vi "Spectrometer Loop.vi"(6 "Used functions":bool, 8 "error in":errorcluster, 9 "Configuration":T1={"Parameter Analizer"={"Parameter Analyzer VISA Session"="COM1", "Sweeping Time Parameters"={"Integration Time"=0, "Short Integration Time (s)"=1.0, "Long Integration Time (s)"=0.0, "Wait Time Parameter"=1.0}, "Acquisition Mode"=enum."Sweeping Mode", "Status Polling Time (ms)"=0, "Comment"="Test VI", "SMU 1 - Sweeping"={"Start / Offset"=0.0, "Stop / Ratio"=1.0, "Step \n(linear only)"=0.01, "Compliance"=0.1, "Power \nCompliance"=0.0, "Mode"=0, "Function"=0, "Sweep Mode"=FALSE}, "SMU 2 - Sweeping"={"Start / Offset"=0.0, "Stop / Ratio"=1.0, "Step \n(linear only)"=0.01, "Compliance"=0.1, "Power \nCompliance"=0.0, "Mode"=0, "Function"=0, "Sweep Mode"=FALSE}, "SMU 3 - Sweeping"={"Start / Offset"=0.0, "Stop / Ratio"=1.0, "Step \n(linear only)"=0.01, "Compliance"=0.1, "Power \nCompliance"=0.0, "Mode"=0, "Function"=0, "Sweep Mode"=FALSE}, "SMU 4 - Sweeping"={"Start / Offset"=0.0, "Stop / Ratio"=1.0, "Step \n(linear only)"=0.01, "Compliance"=0.1, "Power \nCompliance"=0.0, "Mode"=0, "Function"=0, "Sweep Mode"=FALSE}, "Sweep Spacing"=0, "Range"=0, "SMU1 - Sampling"={"Source"=10.0, "Compliance"=1e-05, "Mode"=0, "Function"=FALSE}, "SMU2 - Sampling"={"Source"=1.0, "Compliance"=1.0, "Mode"=0, "Function"=FALSE}, "SMU3 - Sampling"={"Source"=10.0, "Compliance"=1e-05, "Mode"=0, "Function"=FALSE}, "SMU4 - Sampling"={"Source"=0.1, "Compliance"=60.0, "Mode"=10, "Function"=FALSE}, "Sampling Time Parameters"={"Initial Interval (s)"=0.1, "Number of Samples"=60, "Total Sampling Time (s)"=10.0, "Hold Time (s)"=0.0, "Sampling Mode"=0, "Sampling Time"=0}, "Stop Condition"={"Enable Delay (s)"=0.0, "Name"="", "Threshold"=0.0, "num. of events"=1, "Event"=0, "Stop Condition Enable"=FALSE}}, "Switching Matrix"={"Switching Matrix VISA Session"="GPIB0::18::INSTR", "Connections"=[{"Connections"=[FALSE, FALSE, FALSE, FALSE, FALSE, FALSE, FALSE, FALSE, FALSE, FALSE, FALSE, FALSE], "Connection Type"=enum."Disconnected"}, {"Connections"=[FALSE, FALSE, FALSE, FALSE, FALSE, FALSE, FALSE, FALSE, FALSE, FALSE, FALSE, FALSE], "Connection Type"=enum."Disconnected"}, {"Connections"=[FALSE, FALSE, FALSE, FALSE, FALSE, FALSE, FALSE, FALSE, FALSE, FALSE, FALSE, FALSE], "Connection Type"=enum."Disconnected"}, {"Connections"=[FALSE, FALSE, FALSE, FALSE, FALSE, FALSE, FALSE, FALSE, FALSE, FALSE, FALSE, FALSE], "Connection Type"=enum."Disconnected"}, {"Connections"=[FALSE, FALSE, FALSE, FALSE, FALSE, FALSE, FALSE, FALSE, FALSE, FALSE, FALSE, FALSE], "Connection Type"=enum."Disconnected"}, {"Connections"=[FALSE, FALSE, FALSE, FALSE, FALSE, FALSE, FALSE, FALSE, FALSE, FALSE, FALSE, FALSE], "Connection Type"=enum."Disconnected"}, {"Connections"=[FALSE, FALSE, FALSE, FALSE, FALSE, FALSE, FALSE, FALSE, FALSE, FALSE, FALSE, FALSE], "Connection Type"=enum."Disconnected"}, {"Connections"=[FALSE, FALSE, FALSE, FALSE, FALSE, FALSE, FALSE, FALSE, FALSE, FALSE, FALSE, FALSE], "Connection Type"=enum."Disconnected"}]}, "Stress Control"={"Stress Control VISA Session"="StrainMotor", "Axis"=0, "Motion"=0, "Destination (°)"=0.0, "Speed (°/s)"=4.0, "Position (°)"=25.0}, "Optical Spectrometer"={"Laser Settings"={"Laser Wavelength"=enum."365 nm", "Neutral Density Filter"=enum."100%"}, "Spectrometer Settings"={"Confocal Hole Size (µm)"=0.0, "Grating"=2, "Detector"=enum."InGaAs Array"}, "Acquisition Settings"={"Acquisition Mode"=enum."Multi-Window", "Spectal Position (nm)"=632.0, "From (nm)"=735.0, "To (nm)"=0.0, "Integration Time (s)"=0.0, "Number of Accumulations"=3, "AutoScanning"=FALSE, "Spike Removal"=FALSE}, "Path"=path "C:/07 - Prizes and Awards/Marie Curie Prize/Reply Editors Final NCOMMS(10).docx"}, "Switches & Mirrors"={"Relay VISA Session"="COM1", "Switches"={"Laser"=FALSE, "Video"=FALSE}, "Delays (ms)"={"Laser"=500, "Video"=1500}}, "Camera"={"Settings"={"Pixel clock"=20, "Frame rate"=30.0, "Exposure time"=33.21525, "Master Gain"=0, "Red Gain"=0, "Green Gain"=0, "Blue Gain"=0, "Auto Gain"=FALSE, "White-balance"=FALSE, "Color Correction"=FALSE}}, "XYZ Stage"={"Connection Settings"={"Tango VISA"="", "Baudrate"=57600, "Show Protocol?"=FALSE}, "Manual Control"={"North"=FALSE, "South"=FALSE, "West"=FALSE, "East"=FALSE, "Up"=FALSE, "Down"=FALSE, "Stop"=FALSE, "XY Step"=0.0, "Z step"=0.0}, "Coordinate Control"={"Motion Mode"=enum."Absolute", "Destination [mm]"=[]}}, "AutoFocus"={"Matching Criteria"={"Minimum Score"=700.0, "Color Score Weight"=700.0, "Minimum Contrast"=50, "Match Mode"=0, "Match Feature Mode"=0, "Subpixel Accuracy"=TRUE, "Color Sensitivity"=1, "Search Strategy"=1}, "Z Scan Parameters"={"Z Range"=1380.0, "Resolution"=5000.0, "Initial Direction"=enum."Up", "Focus Threshold"=0.1, "Ascent Constant"=0.1}, "Displacement"=0.0, "Transformation Matrix"=[]}, "Sava Data"={"Workspace Info"={"Device Name"="ProberHead_Tst_C29K3_7(2)", "Device Info"="ProberHead_Tst_C29", "Path"=path "C:/Users/gio/Desktop/ProbeHeadTest"}, "Instrument Configuration"={"Instrument"=enum."Unknown Instrument", "Configuration"="Test Configuration"}, "Stress Motor Position"=0.0, "Electrical Measurement"={"Sequence"=[], "V1"=[], "V2"=[], "V3"=[], "V4"=[], "I1"=[], "I2"=[], "I3"=[], "I4"=[]}, "Optical Spectrum"={"Intensity"=[], "Wavelength"=[], "Energy"=[], "Raman Shift"=[], "Detector Temperature"=0.0}}, "PlotData"={"Sliders"={"Strain Sequence"=0, "Instrument Sequence"=0}, "Measurement"={"Which Instrument?"=enum."No Plot", "Electrical Measurement"={"Sequence"=[], "V1"=[], "V2"=[], "V3"=[], "V4"=[], "I1"=[], "I2"=[], "I3"=[], "I4"=[]}, "Measurement Mode"=enum."Sweeping Mode", "Optical Spectrum"={"Intensity"=[], "Wavelength"=[], "Energy"=[], "Raman Shift"=[], "Detector Temperature"=0.0}}, "Instrument Steps"=[], "Strain Points"=[]}, "Instrument Sequence"={"Caller VI"=enum."User"}, "Strain Measurement"={"Stress Sequence "={"Max Motor Position"=1380.0, "# Intermediate Points"=5000, "Initial Direction"=enum."Tension"}, "Track?"=FALSE}} {"AutoFocus"."Displacement" scale=1.0..1000.0; "AutoFocus"."Z Scan Parameters"."Focus Threshold" min=0.0 max=1000.0 step=1.0 format="%#_2f"; "AutoFocus"."Z Scan Parameters"."Ascent Constant" min=0.0 max=1000.0 step=1.0 format="%#_2f"; "AutoFocus"."Z Scan Parameters"."Resolution" min=0.0 max=1.0 step=0.01 format="%_2g"; "AutoFocus"."Z Scan Parameters"."Z Range" format="%_3g"; "AutoFocus"."Matching Criteria"."Match Mode" items=["Shift Invariant", "Rotation Invariant"]; "AutoFocus"."Matching Criteria"."Match Feature Mode" items=["Color and Shape", "Color", "Shape"]; "AutoFocus"."Matching Criteria"."Color Sensitivity" items=["Low Sensitivity", "Medium Sensitivity", "High Sensitivity"]; "AutoFocus"."Matching Criteria"."Search Strategy" items=["Conservative", "Balance", "Aggressive", "Very Aggressive"]; "XYZ Stage"."Manual Control"."Z step" scale=0.1..10.0; "XYZ Stage"."Manual Control"."XY Step" scale=0.1..1000.0; "Camera"."Settings"."Blue Gain" min=0 max=100 scale=0.0..100.0; "Camera"."Settings"."Green Gain" min=0 max=100 scale=0.0..100.0; "Camera"."Settings"."Red Gain" min=0 max=100 scale=0.0..100.0; "Camera"."Settings"."Master Gain" min=0 max=100 scale=0.0..100.0; "Camera"."Settings"."Exposure time" min=0.101625 max=159.246375 step=0.101625 scale=0.101625..159.246375 scale format="%#.3g"; "Camera"."Settings"."Frame rate" min=2.7455631699174137 max=6.2675785993528725 step=0.000101625 scale=2.7455631699174137..6.2675785993528725 scale format="%^#_3g"; "Camera"."Settings"."Pixel clock" min=5 max=43 scale=5.0..43.0; "PlotData"."Sliders"."Instrument Sequence" scale=0.0..10.0; "PlotData"."Sliders"."Strain Sequence" scale=0.0..10.0; "Strain Measurement"."Stress Sequence"."# Intermediate Points" max=1390; "Parameter Analizer"."Stop Condition"."Event" items=["Value > Threshold", "Value < Threshold", "| Value | > | Threshold |", "| Value | < | Threshold |"]; "Parameter Analizer"."Stop Condition"."Threshold" format="%^.2e"; "Parameter Analizer"."Stop Condition"."Enable Delay (s)" format="%.1f"; "Parameter Analizer"."Sampling Time Parameters"."Sampling Time" items=["Auto (linear only)", "No Limit", "Set Limit"]; "Parameter Analizer"."Sampling Time Parameters"."Sampling Mode" items=["Linear", "Log10", "Log25", "Log50", "Thinned Out"]; "Parameter Analizer"."Sampling Time Parameters"."Hold Time (s)" format="%.4f"; "Parameter Analizer"."Sampling Time Parameters"."Total Sampling Time (s)" format="%.1f"; "Parameter Analizer"."Sampling Time Parameters"."Initial Interval (s)" format="%^.3e"; "Parameter Analizer"."SMU 4 - Sweeping"."Function" items=["Disabled", "Var 1", "Var 2", "Var 1'", "Constant"]; "Parameter Analizer"."SMU 4 - Sweeping"."Mode" items=["V", "I", "V pulse", "I  pulse", "Common"]; "Parameter Analizer"."SMU 4 - Sweeping"."Power \nCompliance" format="%^.2e"; "Parameter Analizer"."SMU 4 - Sweeping"."Compliance" format="%^.2e"; "Parameter Analizer"."SMU 4 - Sweeping"."Step \n(linear only)" format="%^.4e"; "Parameter Analizer"."SMU 4 - Sweeping"."Stop / Ratio" format="%^.4e"; "Parameter Analizer"."SMU 4 - Sweeping"."Start / Offset" format="%^.4e"; "Parameter Analizer"."SMU 3 - Sweeping"."Function" items=["Disabled", "Var 1", "Var 2", "Var 1'", "Constant"]; "Parameter Analizer"."SMU 3 - Sweeping"."Mode" items=["V", "I", "V pulse", "I  pulse", "Common"]; "Parameter Analizer"."SMU 3 - Sweeping"."Power \nCompliance" format="%^.2e"; "Parameter Analizer"."SMU 3 - Sweeping"."Compliance" format="%^.2e"; "Parameter Analizer"."SMU 3 - Sweeping"."Step \n(linear only)" format="%^.4e"; "Parameter Analizer"."SMU 3 - Sweeping"."Stop / Ratio" format="%^.4e"; "Parameter Analizer"."SMU 3 - Sweeping"."Start / Offset" format="%^.4e"; "Parameter Analizer"."SMU 2 - Sweeping"."Function" items=["Disabled", "Var 1", "Var 2", "Var 1'", "Constant"]; "Parameter Analizer"."SMU 2 - Sweeping"."Mode" items=["V", "I", "V pulse", "I  pulse", "Common"]; "Parameter Analizer"."SMU 2 - Sweeping"."Power \nCompliance" format="%^.2e"; "Parameter Analizer"."SMU 2 - Sweeping"."Compliance" format="%^.2e"; "Parameter Analizer"."SMU 2 - Sweeping"."Step \n(linear only)" format="%^.4e"; "Parameter Analizer"."SMU 2 - Sweeping"."Stop / Ratio" format="%^.4e"; "Parameter Analizer"."SMU 2 - Sweeping"."Start / Offset" format="%^.4e"; "Parameter Analizer"."SMU 1 - Sweeping"."Function" items=["Disabled", "Var 1", "Var 2", "Var 1'", "Constant"]; "Parameter Analizer"."SMU 1 - Sweeping"."Mode" items=["V", "I", "V pulse", "I  pulse", "Common"]; "Parameter Analizer"."SMU 1 - Sweeping"."Power \nCompliance" format="%^.2e"; "Parameter Analizer"."SMU 1 - Sweeping"."Compliance" format="%^.2e"; "Parameter Analizer"."SMU 1 - Sweeping"."Step \n(linear only)" format="%^.4e"; "Parameter Analizer"."SMU 1 - Sweeping"."Stop / Ratio" format="%^.4e"; "Parameter Analizer"."SMU 1 - Sweeping"."Start / Offset" format="%^.4e"; "Parameter Analizer"."Sweeping Time Parameters"."Long Integration Time (s)" scale=0.02..2.0; "Parameter Analizer"."Sweeping Time Parameters"."Short Integration Time (s)" scale=8e-05..0.00192; "Parameter Analizer"."Sweeping Time Parameters"."Integration Time" items=["Short", "Long"]; "Parameter Analizer"."Sweeping Time Parameters"."Wait Time Parameter" format="%.1f"; "Parameter Analizer"."SMU4 - Sampling"."Mode" items=["V", "I", "Common"]; "Parameter Analizer"."SMU4 - Sampling"."Compliance" format="%^.2e"; "Parameter Analizer"."SMU4 - Sampling"."Source" format="%^.3e"; "Parameter Analizer"."SMU3 - Sampling"."Mode" items=["V", "I", "Common"]; "Parameter Analizer"."SMU3 - Sampling"."Compliance" format="%^.2e"; "Parameter Analizer"."SMU3 - Sampling"."Source" format="%^.3e"; "Parameter Analizer"."SMU2 - Sampling"."Mode" items=["V", "I", "Common"]; "Parameter Analizer"."SMU2 - Sampling"."Compliance" format="%^.2e"; "Parameter Analizer"."SMU2 - Sampling"."Source" format="%^.3e"; "Parameter Analizer"."SMU1 - Sampling"."Mode" items=["V", "I", "Common"]; "Parameter Analizer"."SMU1 - Sampling"."Compliance" format="%^.2e"; "Parameter Analizer"."SMU1 - Sampling"."Source" format="%^.3e"; "Parameter Analizer"."Range" items=["auto", "fixed", "limited"]; "Parameter Analizer"."Sweep Spacing" items=["linear", "log 10", "log 25", "log 50"]; "Stress Control"."Axis" min=1 max=3; "Stress Control"."Position (°)" format="%.6g"; "Stress Control"."Speed (°/s)" min=0.0 max=4.0 format="%.6f"; "Stress Control"."Destination (°)" min=-2000000000.0 max=2000000000.0 format="%.6f"; "Stress Control"."Motion" items=["Absolute", "Relative"]; "Optical Spectrometer"."Spectrometer Settings"."Grating" items=["1800 l/mm", "150 l/mm"]}, 10 "Message Queues out":T57, 11 "Notifiers":T44) -> (0 "error out":errorcluster)   [LabVIEW 2014]
uses:
  support/Message Queue/All Message Queues.ctl
  support/Message Queue/Message Cluster.ctl
  support/Notifiers/Notifiers.ctl
  support/Message Handler Loop Notifiers.ctl
  Hardware Control/Parameter Analyzer/Parameter Analyzer Notifiers.ctl
  Hardware Control/Switching Matrix/Switching Matrix Notifiers.ctl
  Hardware Control/Stress Control/StressControl Notifiers.ctl
  Hardware Control/Spectrometer/Spectrometer Notifiers.ctl
  Hardware Control/Switches and Mirrors/SwitchesMirrors Notifiers.ctl
  Hardware Control/Camera/Camera Notifiers.ctl
  Hardware Control/XYZ Stage/XYZ Notifications.ctl
  Hardware Control/Autofocus/Autofocus Notifiers.ctl
  Measurements/Optoelectronic Measurement/Optoelectronic Notifiers.ctl
  Measurements/Save Data/SaveData Notifiers.ctl
  Measurements/Instrument Sequence/Instrument Sequence Notifiers.ctl
  support/Configuration/Configuration.ctl
  Hardware Control/Parameter Analyzer/Parameter Analyzer Config.ctl
  Hardware Control/Parameter Analyzer/Parameter Analyzer Integration Parameters.ctl
  Hardware Control/Parameter Analyzer/Parameter Analyzer SMU Sweeping.ctl
  Hardware Control/Parameter Analyzer/Parameter Analyzer Sweep Spacing.ctl
  Hardware Control/Parameter Analyzer/Parameter Analyzer SMU Range.ctl
  Hardware Control/Parameter Analyzer/Parameter Analyzer SMU Sampling.ctl
  Hardware Control/Parameter Analyzer/Parameter Analyzer Sampling Parameters.ctl
  Hardware Control/Parameter Analyzer/Parameter Analyzer Stop Sampling Conditions.ctl
  Hardware Control/Switching Matrix/Switching Matrix Config.ctl
  Hardware Control/Stress Control/StressControl Config.ctl
  Hardware Control/Spectrometer/Spectrometer Config.ctl
  Hardware Control/Spectrometer/Laser Settings.ctl
  Hardware Control/Spectrometer/Laser.ctl
  Hardware Control/Spectrometer/Filter.ctl
  Hardware Control/Spectrometer/Grating Detector Settings.ctl
  Hardware Control/Spectrometer/Grating.ctl
  Hardware Control/Spectrometer/Detector.ctl
  Hardware Control/Spectrometer/Acquisition Settings.ctl
  Hardware Control/Switches and Mirrors/SwitchesMirrors Config.ctl
  Hardware Control/Switches and Mirrors/SwitchesMirrors Status.ctl
  Hardware Control/Camera/Camera Config.ctl
  Hardware Control/Camera/Camera Settings.ctl
  Hardware Control/XYZ Stage/XYZ Config.ctl
  Hardware Control/XYZ Stage/XYZ Connection Settings.ctl
  Hardware Control/XYZ Stage/XYZ Stage Control.ctl
  Hardware Control/XYZ Stage/XYZ Coordinate Control.ctl
  Hardware Control/Autofocus/AutoFocus Config.ctl
  Hardware Control/Autofocus/ZScan.ctl
  <vilib>/Analysis/Matrix/Datatypes/RealMatrix.ctl
  Measurements/Save Data/SaveData Config.ctl
  Measurements/Save Data/SaveData Workspace Info.ctl
  Measurements/Save Data/SaveData Instrument Configuration.ctl
  Measurements/Instrument Sequence/Instrument List.ctl
  Hardware Control/Spectrometer/Spectral Data.ctl
  Measurements/Plot Data/PlotData Config.ctl
  Measurements/Plot Data/Measurement.ctl
  Measurements/Plot Data/WhichInstrument.ctl
  Hardware Control/Parameter Analyzer/Electrical Data.ctl
  Measurements/Instrument Sequence/Instrument Steps.ctl
  Measurements/Instrument Sequence/Action.ctl
  Measurements/Instrument Sequence/Instrument Sequence Config.ctl
  Measurements/Strain Measurement/Strain Measurement Config.ctl
  Hardware Control/Spectrometer/Spectrometer Function.ctl
  support/Message Queue/Enqueue Message (Array).vi
  support/Message Queue/Message Queue.lvlib
  <vilib>/Analysis/Matrix/NI_Matrix.lvlib
panel:
  # "LICENSED MATERIALS – PROPERTY OF IBM\nCopyright IBM Corp. 2016,\nALL RIGHTS RESERVED"
  # "XY"
  # "Z"
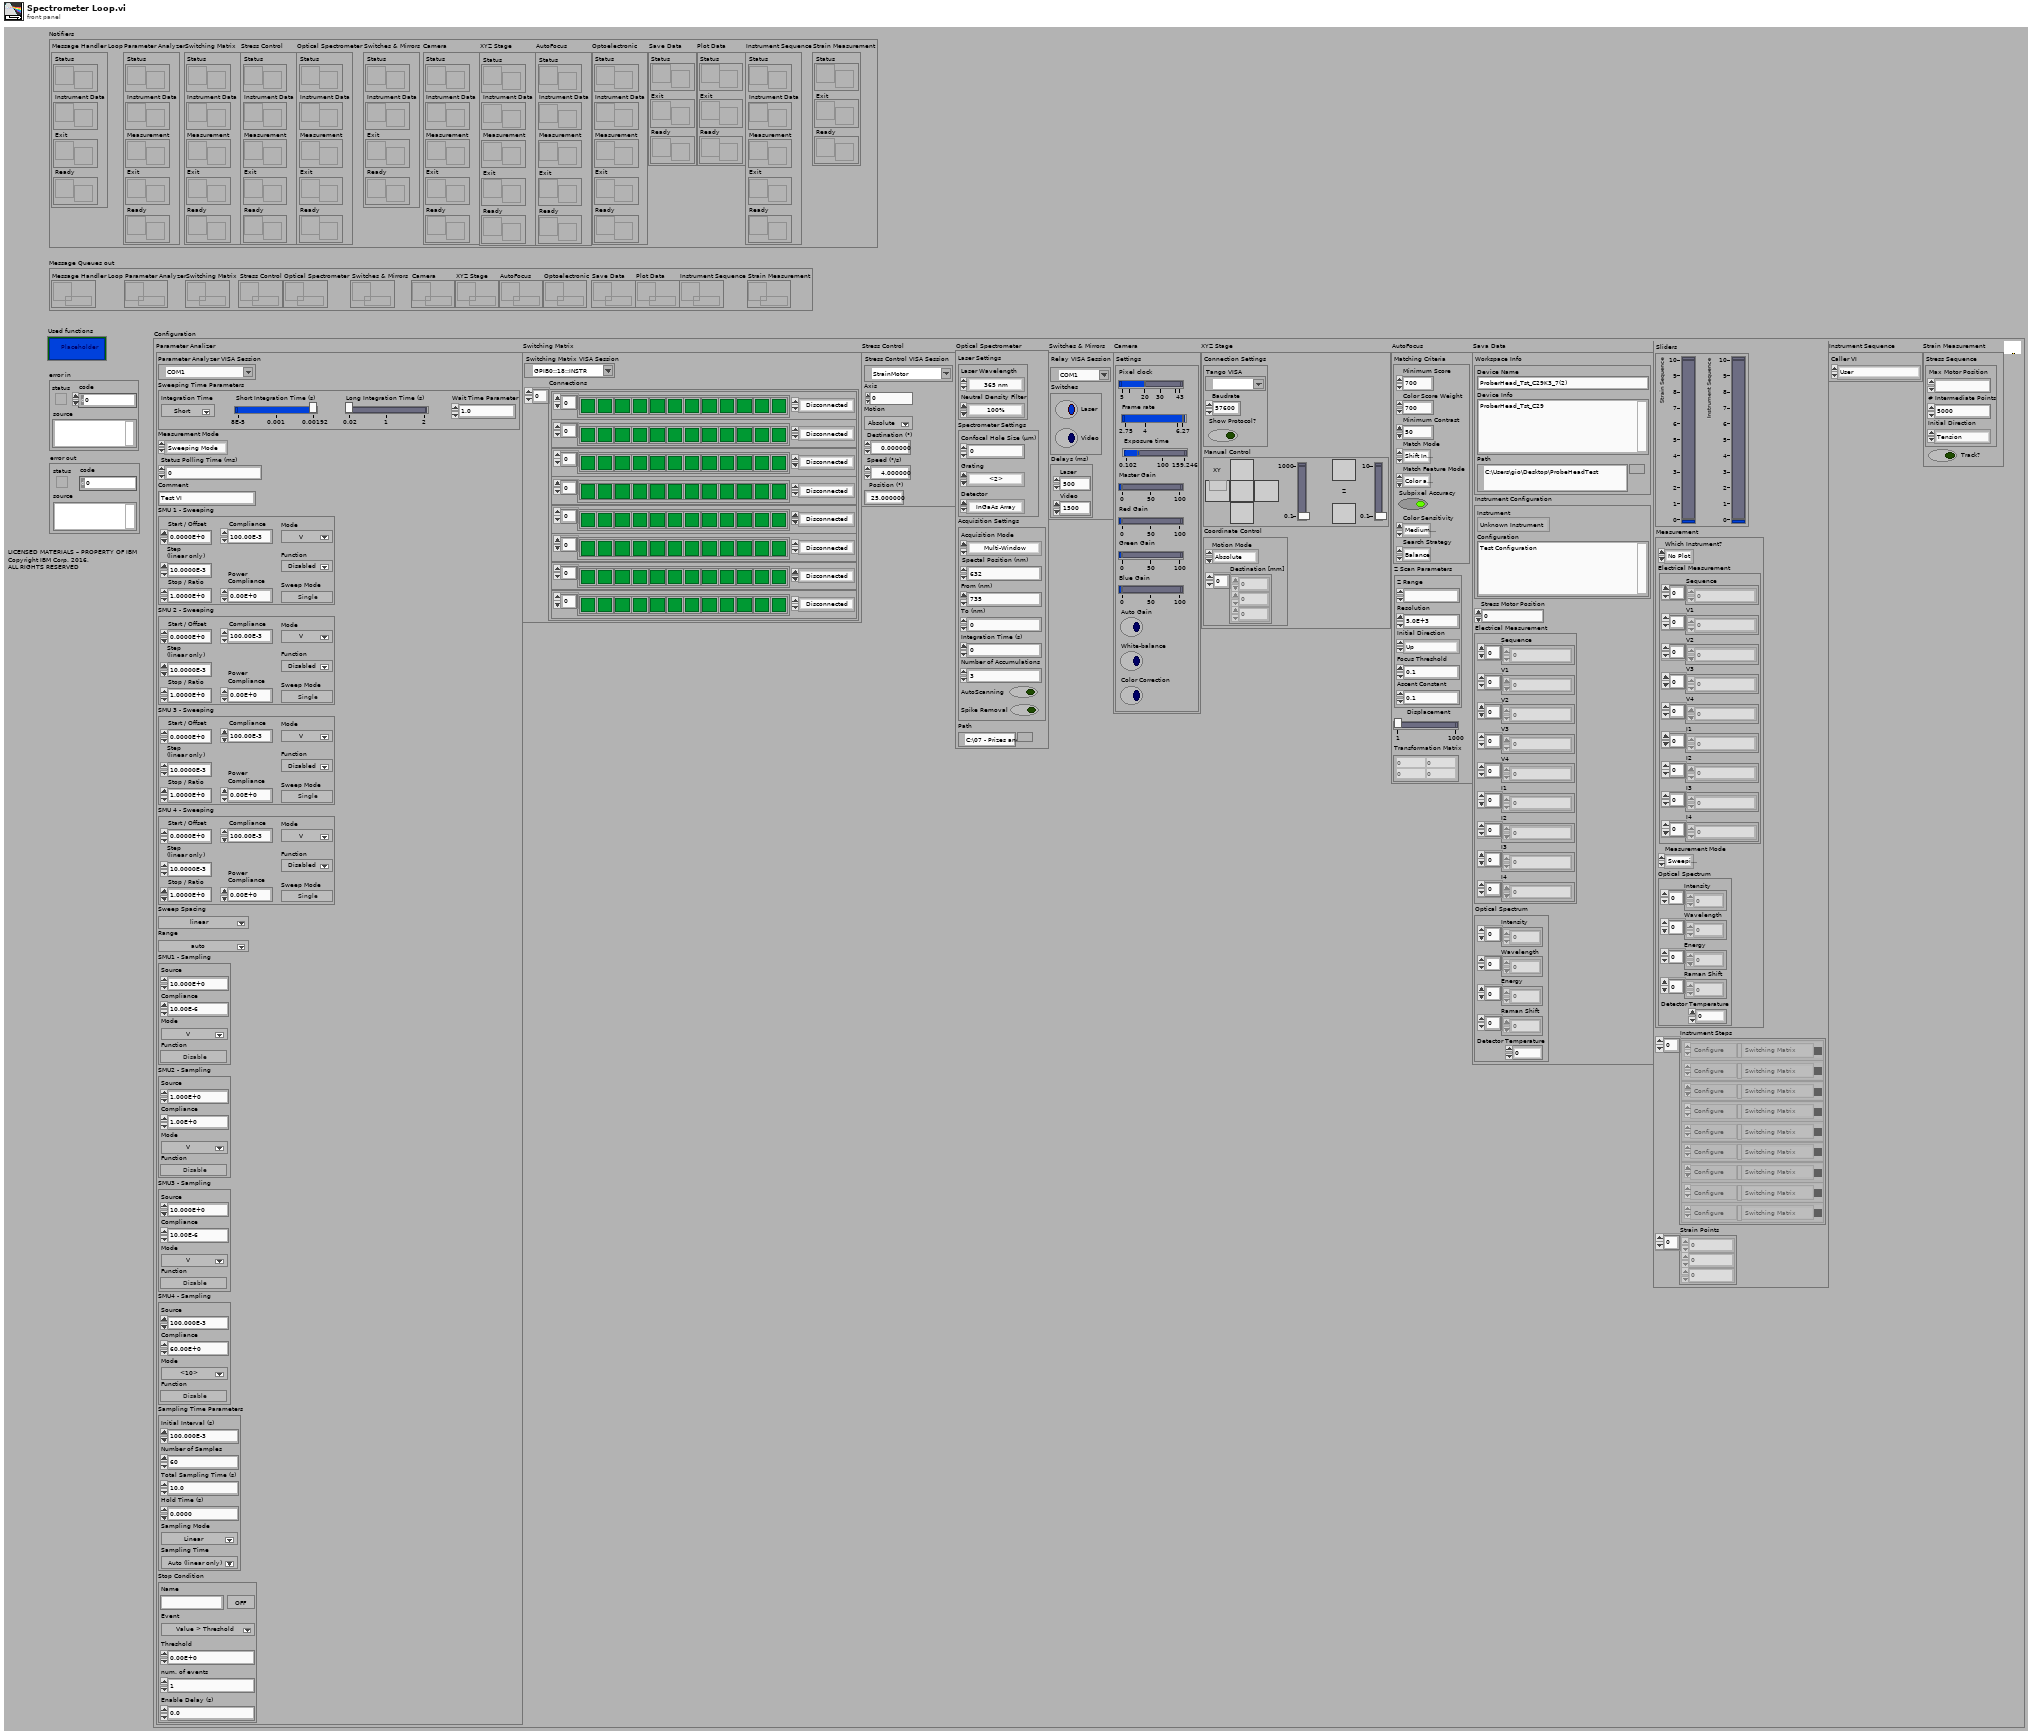
[diagram p1: front panel]
types:
  T1 = typedef "Configuration.ctl" = cluster{"Parameter Analizer":T2, "Switching Matrix":T10, "Stress Control":T11, "Optical Spectrometer":T12, "Switches & Mirrors":T20, "Camera":T22, "XYZ Stage":T24, "AutoFocus":T28, "Sava Data":T31, "PlotData":T36, "Instrument Sequence":T42, "Strain Measurement":T43}
  T2 = typedef "Parameter Analyzer Config.ctl" = cluster{"Parameter Analyzer VISA Session":refnum<visa-resource-name>, "Sweeping Time Parameters":T3, "Acquisition Mode":enum32{"Sweeping Mode", "Sampling Mode"}, "Status Polling Time (ms)":u32, "Comment":string, "SMU 1 - Sweeping":T4, "SMU 2 - Sweeping":T4, "SMU 3 - Sweeping":T4, "SMU 4 - Sweeping":T4, "Sweep Spacing":T5, "Range":T6, "SMU1 - Sampling":T7, "SMU2 - Sampling":T7, "SMU3 - Sampling":T7, "SMU4 - Sampling":T7, "Sampling Time Parameters":T8, "Stop Condition":T9}
  T3 = typedef "Parameter Analyzer Integration Parameters.ctl" = cluster{"Integration Time":u32, "Short Integration Time (s)":dbl, "Long Integration Time (s)":dbl, "Wait Time Parameter":dbl}
  T4 = typedef "Parameter Analyzer SMU Sweeping.ctl" = cluster{"Start / Offset":dbl, "Stop / Ratio":dbl, "Step \n(linear only)":dbl, "Compliance":dbl, "Power \nCompliance":dbl, "Mode":u32, "Function":i32, "Sweep Mode":bool}
  T5 = typedef "Parameter Analyzer Sweep Spacing.ctl" = u16
  T6 = typedef "Parameter Analyzer SMU Range.ctl" = u16
  T7 = typedef "Parameter Analyzer SMU Sampling.ctl" = cluster{"Source":dbl, "Compliance":dbl, "Mode":u32, "Function":bool}
  T8 = typedef "Parameter Analyzer Sampling Parameters.ctl" = cluster{"Initial Interval (s)":dbl, "Number of Samples":i32, "Total Sampling Time (s)":dbl, "Hold Time (s)":dbl, "Sampling Mode":i32, "Sampling Time":i32}
  T9 = typedef "Parameter Analyzer Stop Sampling Conditions.ctl" = cluster{"Enable Delay (s)":dbl, "Name":string, "Threshold":dbl, "num. of events":i32, "Event":i32, "Stop Condition Enable":bool}
  T10 = typedef "Switching Matrix Config.ctl" = cluster{"Switching Matrix VISA Session":refnum<visa-resource-name>, "Connections":cluster{"Connections":bool[], "Connection Type":enum16{"Disconnected", "Make - Break", "Break - Make"}}[]}
  T11 = typedef "StressControl Config.ctl" = cluster{"Stress Control VISA Session":refnum<visa-resource-name>, "Axis":i32, "Motion":u16, "Destination (°)":dbl, "Speed (°/s)":dbl, "Position (°)":dbl}
  T12 = typedef "Spectrometer Config.ctl" = cluster{"Laser Settings":T13, "Spectrometer Settings":T16, "Acquisition Settings":T19, "Path":path}
  T13 = typedef "Laser Settings.ctl" = cluster{"Laser Wavelength":T14, "Neutral Density Filter":T15}
  T14 = typedef "Laser.ctl" = enum16{"633 nm", "784 nm", "532 nm", "365 nm"}
  T15 = typedef "Filter.ctl" = enum16{"100%", "50%", "25%", "10%", "1%", "0.1%", "0.01%"}
  T16 = typedef "Grating Detector Settings.ctl" = cluster{"Confocal Hole Size (µm)":dbl, "Grating":T17, "Detector":T18}
  T17 = typedef "Grating.ctl" = u16
  T18 = typedef "Detector.ctl" = enum16{"InGaAs Array", "Silicon CCD"}
  T19 = typedef "Acquisition Settings.ctl" = cluster{"Acquisition Mode":enum16{"Single Window", "Multi-Window"}, "Spectal Position (nm)":dbl, "From (nm)":dbl, "To (nm)":dbl, "Integration Time (s)":dbl, "Number of Accumulations":i32, "AutoScanning":bool, "Spike Removal":bool}
  T20 = typedef "SwitchesMirrors Config.ctl" = cluster{"Relay VISA Session":refnum<visa-resource-name>, "Switches":T21, "Delays (ms)":cluster{"Laser":u32, "Video":u32}}
  T21 = typedef "SwitchesMirrors Status.ctl" = cluster{"Laser":bool, "Video":bool}
  T22 = typedef "Camera Config.ctl" = cluster{"Settings":T23}
  T23 = typedef "Camera Settings.ctl" = cluster{"Pixel clock":i32, "Frame rate":dbl, "Exposure time":dbl, "Master Gain":i32, "Red Gain":i32, "Green Gain":i32, "Blue Gain":i32, "Auto Gain":bool, "White-balance":bool, "Color Correction":bool}
  T24 = typedef "XYZ Config.ctl" = cluster{"Connection Settings":T25, "Manual Control":T26, "Coordinate Control":T27}
  T25 = typedef "XYZ Connection Settings.ctl" = cluster{"Tango VISA":refnum<visa-resource-name>, "Baudrate":i32, "Show Protocol?":bool}
  T26 = typedef "XYZ Stage Control.ctl" = cluster{"North":bool, "South":bool, "West":bool, "East":bool, "Up":bool, "Down":bool, "Stop":bool, "XY Step":dbl, "Z step":dbl}
  T27 = typedef "XYZ Coordinate Control.ctl" = cluster{"Motion Mode":enum16{"Absolute", "Relative"}, "Destination [mm]":dbl[]}
  T28 = typedef "AutoFocus Config.ctl" = cluster{"Matching Criteria":cluster{"Minimum Score":sgl, "Color Score Weight":sgl, "Minimum Contrast":i32, "Match Mode":u32, "Match Feature Mode":u32, "Subpixel Accuracy":bool, "Color Sensitivity":u32, "Search Strategy":u32}, "Z Scan Parameters":T29, "Displacement":dbl, "Transformation Matrix":T30}
  T29 = typedef "ZScan.ctl" = cluster{"Z Range":ext, "Resolution":dbl, "Initial Direction":enum16{"Up", "Down"}, "Focus Threshold":dbl, "Ascent Constant":dbl}
  T30 = typedef "NI_Matrix.lvlib/RealMatrix.ctl" = dbl[][]
  T31 = typedef "SaveData Config.ctl" = cluster{"Workspace Info":T32, "Instrument Configuration":T33, "Stress Motor Position":dbl, "Electrical Measurement":cluster{"Sequence":dbl[], "V1":dbl[], "V2":dbl[], "V3":dbl[], "V4":dbl[], "I1":dbl[], "I2":dbl[], "I3":dbl[], "I4":dbl[]}, "Optical Spectrum":T35}
  T32 = typedef "SaveData Workspace Info.ctl" = cluster{"Device Name":string, "Device Info":string, "Path":path}
  T33 = typedef "SaveData Instrument Configuration.ctl" = cluster{"Instrument":T34, "Configuration":string}
  T34 = typedef "Instrument List.ctl" = enum32{"Unknown Instrument", "Switching Matrix", "Parameter Analyzer", "Optical Spectrometer", "Optoelectronic", "Autofocus"}
  T35 = typedef "Spectral Data.ctl" = cluster{"Intensity":dbl[], "Wavelength":dbl[], "Energy":dbl[], "Raman Shift":dbl[], "Detector Temperature":dbl}
  T36 = typedef "PlotData Config.ctl" = cluster{"Sliders":cluster{"Strain Sequence":i32, "Instrument Sequence":i32}, "Measurement":T37, "Instrument Steps":T40, "Strain Points":dbl[]}
  T37 = typedef "Measurement.ctl" = cluster{"Which Instrument?":T38, "Electrical Measurement":T39, "Measurement Mode":enum16{"Sweeping Mode", "Sampling Mode"}, "Optical Spectrum":T35}
  T38 = typedef "WhichInstrument.ctl" = enum16{"No Plot", "Spectrometer", "Parameter Analyzer", "Optoelectronic"}
  T39 = typedef "Electrical Data.ctl" = cluster{"Sequence":dbl[], "V1":dbl[], "V2":dbl[], "V3":dbl[], "V4":dbl[], "I1":dbl[], "I2":dbl[], "I3":dbl[], "I4":dbl[]}
  T40 = typedef "Instrument Steps.ctl" = cluster{"Action":T41, "Configuration":variant, "Instrument":T34, "Status":enum8{"False", "True", "Mixed"}}[]
  T41 = typedef "Action.ctl" = enum32{"Configure", "Measure"}
  T42 = typedef "Instrument Sequence Config.ctl" = cluster{"Caller VI":enum16{"User", "Stress Measurement VI"}}
  T43 = typedef "Strain Measurement Config.ctl" = cluster{"Stress Sequence ":cluster{"Max Motor Position":ext, "# Intermediate Points":u32, "Initial Direction":enum16{"Tension", "Compression"}}, "Track?":bool}
  T44 = typedef "Notifiers.ctl" = cluster{"Message Handler Loop":T45, "Parameter Analyzer":T46, "Switching Matrix":T47, "Stress Control":T48, "Optical Spectrometer":T49, "Switches & Mirrors":T50, "Camera":T51, "XYZ Stage":T52, "AutoFocus":T53, "Optoelectronic":T54, "Save Data":T55, "Plot Data":T55, "Instrument Sequence":T56, "Strain Measurement":cluster{"Status":refnum<notifier>, "Exit":refnum<notifier>, "Ready":refnum<notifier>}}
  T45 = typedef "Message Handler Loop Notifiers.ctl" = cluster{"Status":refnum<notifier>, "Instrument Data":refnum<notifier>, "Exit":refnum<notifier>, "Ready":refnum<notifier>}
  T46 = typedef "Parameter Analyzer Notifiers.ctl" = cluster{"Status":refnum<notifier>, "Instrument Data":refnum<notifier>, "Measurement":refnum<notifier>, "Exit":refnum<notifier>, "Ready":refnum<notifier>}
  T47 = typedef "Switching Matrix Notifiers.ctl" = cluster{"Status":refnum<notifier>, "Instrument Data":refnum<notifier>, "Measurement":refnum<notifier>, "Exit":refnum<notifier>, "Ready":refnum<notifier>}
  T48 = typedef "StressControl Notifiers.ctl" = cluster{"Status":refnum<notifier>, "Instrument Data":refnum<notifier>, "Measurement":refnum<notifier>, "Exit":refnum<notifier>, "Ready":refnum<notifier>}
  T49 = typedef "Spectrometer Notifiers.ctl" = cluster{"Status":refnum<notifier>, "Instrument Data":refnum<notifier>, "Measurement":refnum<notifier>, "Exit":refnum<notifier>, "Ready":refnum<notifier>}
  T50 = typedef "SwitchesMirrors Notifiers.ctl" = cluster{"Status":refnum<notifier>, "Instrument Data":refnum<notifier>, "Exit":refnum<notifier>, "Ready":refnum<notifier>}
  T51 = typedef "Camera Notifiers.ctl" = cluster{"Status":refnum<notifier>, "Instrument Data":refnum<notifier>, "Measurement":refnum<notifier>, "Exit":refnum<notifier>, "Ready":refnum<notifier>}
  T52 = typedef "XYZ Notifications.ctl" = cluster{"Status":refnum<notifier>, "Instrument Data":refnum<notifier>, "Measurement":refnum<notifier>, "Exit":refnum<notifier>, "Ready":refnum<notifier>}
  T53 = typedef "Autofocus Notifiers.ctl" = cluster{"Status":refnum<notifier>, "Instrument Data":refnum<notifier>, "Measurement":refnum<notifier>, "Exit":refnum<notifier>, "Ready":refnum<notifier>}
  T54 = typedef "Optoelectronic Notifiers.ctl" = cluster{"Status":refnum<notifier>, "Instrument Data":refnum<notifier>, "Measurement":refnum<notifier>, "Exit":refnum<notifier>, "Ready":refnum<notifier>}
  T55 = typedef "SaveData Notifiers.ctl" = cluster{"Status":refnum<notifier>, "Exit":refnum<notifier>, "Ready":refnum<notifier>}
  T56 = typedef "Instrument Sequence Notifiers.ctl" = cluster{"Status":refnum<notifier>, "Instrument Data":refnum<notifier>, "Measurement":refnum<notifier>, "Exit":refnum<notifier>, "Ready":refnum<notifier>}
  T57 = typedef "Message Queue.lvlib/All Message Queues.ctl" = cluster{"Message Handler Loop":refnum<queue>, "Parameter Analyzer":refnum<queue>, "Switching Matrix":refnum<queue>, "Stress Control":refnum<queue>, "Optical Spectrometer":refnum<queue>, "Switches & Mirrors":refnum<queue>, "Camera":refnum<queue>, "XYZ Stage":refnum<queue>, "AutoFocus":refnum<queue>, "Optoelectronic":refnum<queue>, "Save Data":refnum<queue>, "Plot Data":refnum<queue>, "Instrument Sequence":refnum<queue>, "Strain Measurement":refnum<queue>}
  T58 = typedef "Spectrometer Data.ctl" = cluster{"Configuration":T12, "Refnums":T59, "Initialization":T61}
  T59 = typedef "Spectrometer Refnum.ctl" = cluster{"Instrument Status":refnum<vi>, "Optical Spectrum Plot":T60, "Laser":refnum<vi>, "Filter":refnum<vi>, "Laser ON?":refnum<vi>, "Hole":refnum<vi>, "Grating":refnum<vi>, "Detector":refnum<vi>, "Acquisition Mode":refnum<vi>, "Spectal Position":refnum<vi>, "From":refnum<vi>, "To":refnum<vi>, "Integration Time":refnum<vi>, "Accumulations":refnum<vi>, "AutoScanning":refnum<vi>, "Spike Removal":refnum<vi>, "Acquisition Mode Panel":refnum<vi>}
  T60 = typedef "Optical Spectrum Plot Refnum.ctl" = cluster{"Plot List":refnum<vi>, "Optical Spectrum vs Energy":refnum<vi>, "Optical Spectrum vs Wavelength":refnum<vi>, "Optical Spectrum vs Raman Shift":refnum<vi>, "Detector Temperature":refnum<vi>}
  T61 = typedef "Spectrometer Initialization.ctl" = cluster{"Connect":bool, "Update Refnums":bool, "Get Configuration":bool}
  T62 = typedef "Spectrometer Function.ctl" = enum16{"Connect", "Complete Configuration", "Get Status", "Load Configuration", "Save Configuration", "Acquire Spectrum", "Read File", "Set Laser", "Set Filter", "Set Hole", "Set Grating", "Set Grating Position", "Set Detector", "Set Acquisition Mode", "Update Refnums", "Disconnect"}
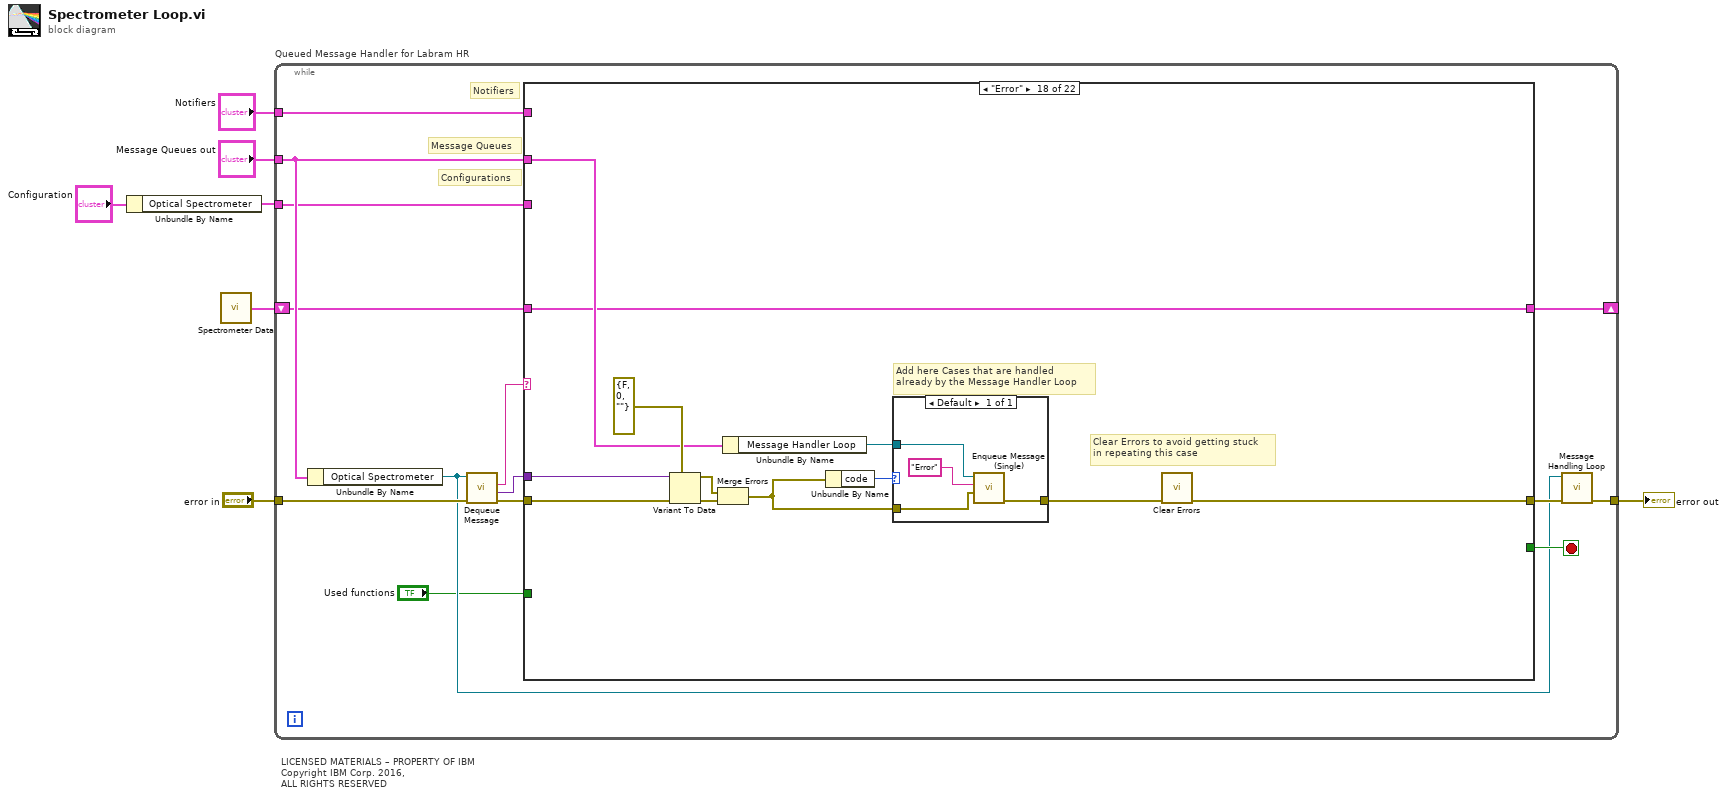
[diagram p0: block diagram]
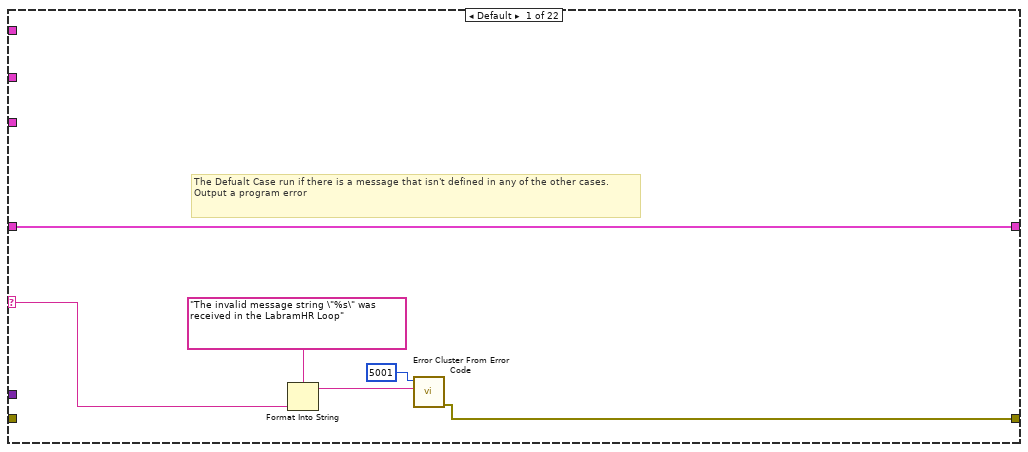
[diagram p2: hidden frame]
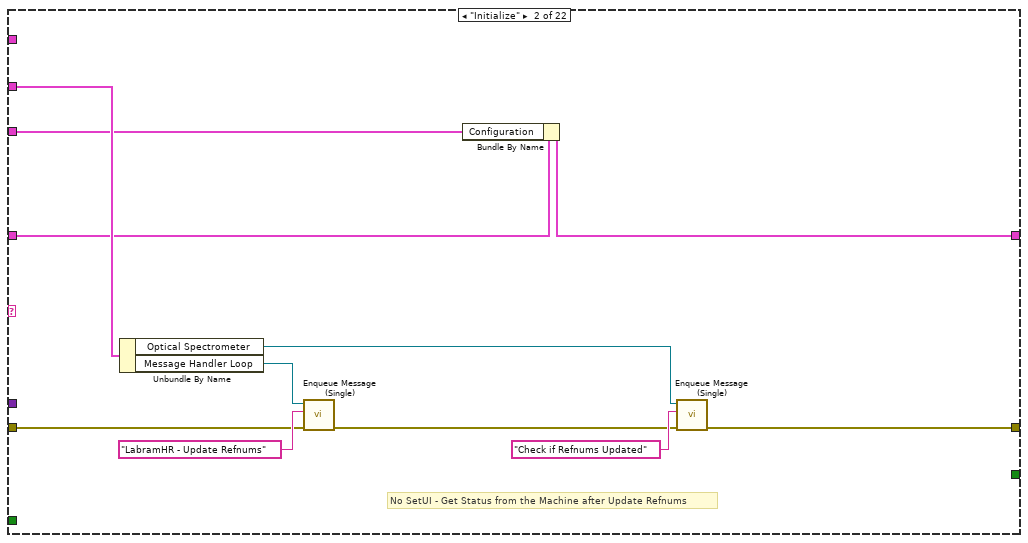
[diagram p3: hidden frame]
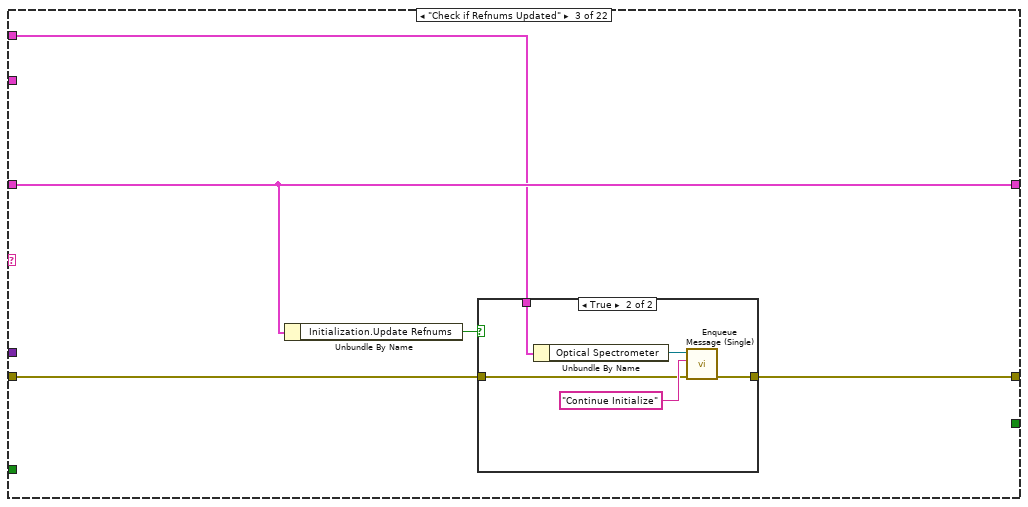
[diagram p4: hidden frame]
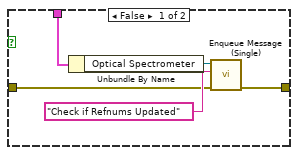
[diagram p5: hidden frame]
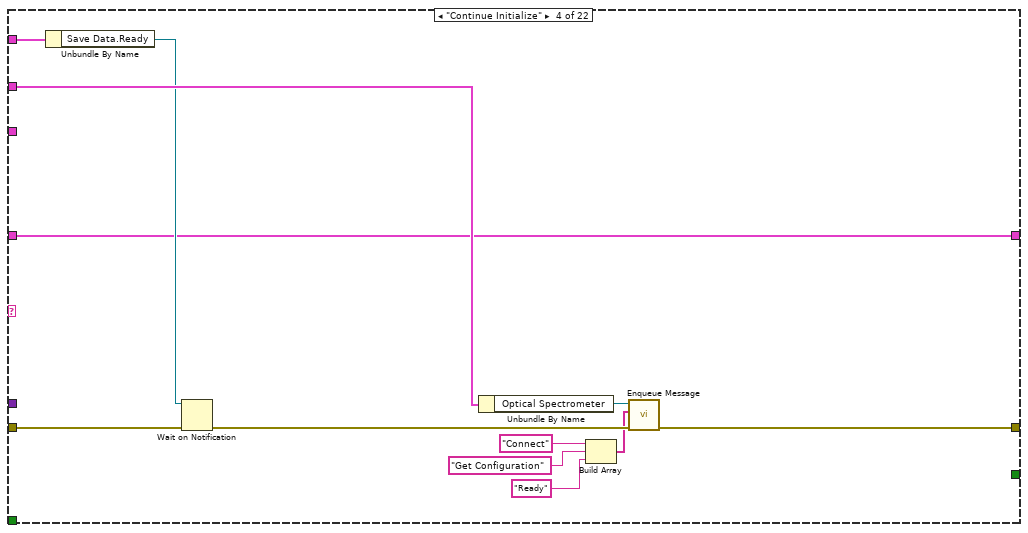
[diagram p6: hidden frame]
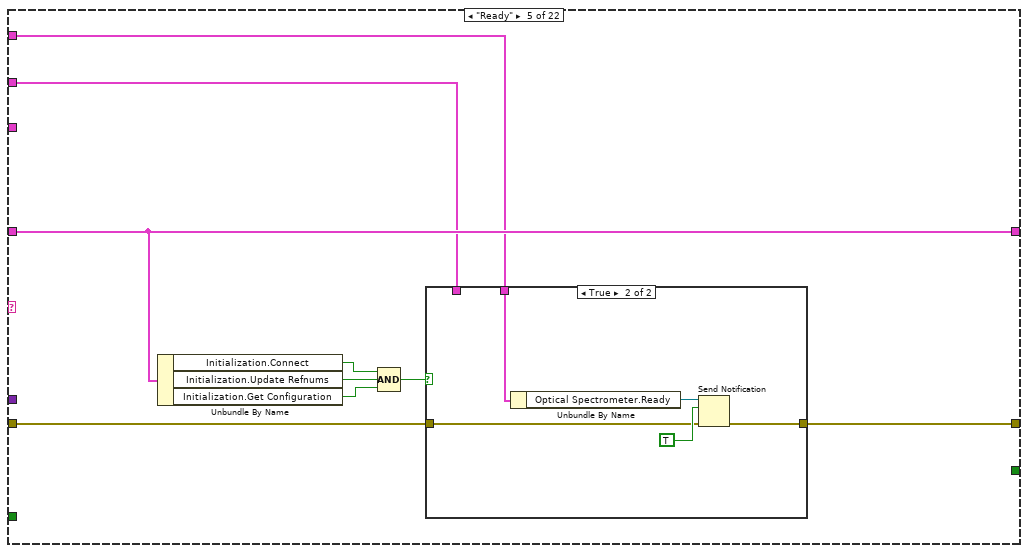
[diagram p7: hidden frame]
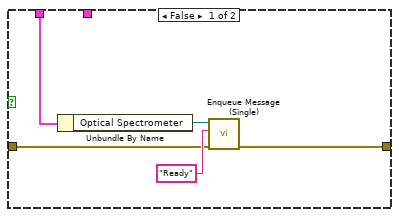
[diagram p8: hidden frame]
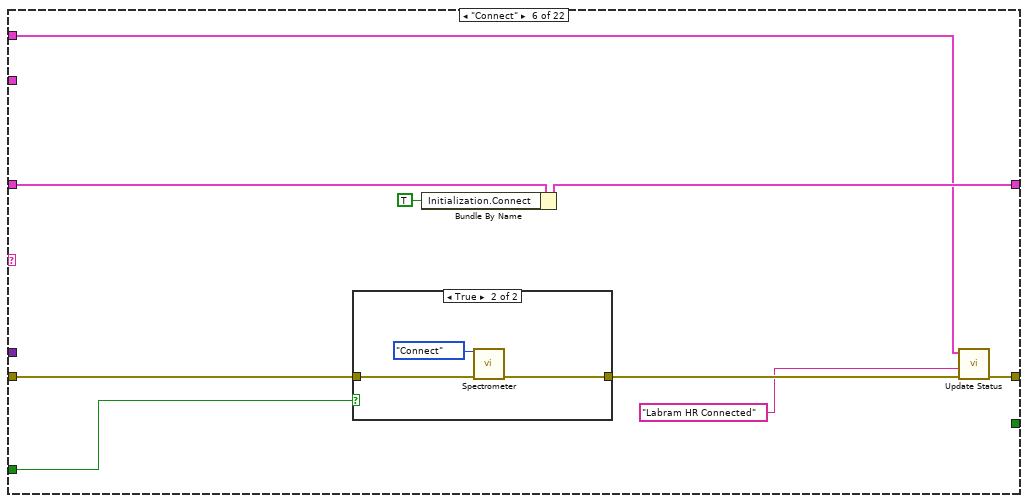
[diagram p9: hidden frame]
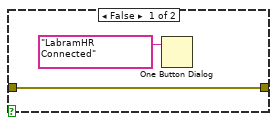
[diagram p10: hidden frame]
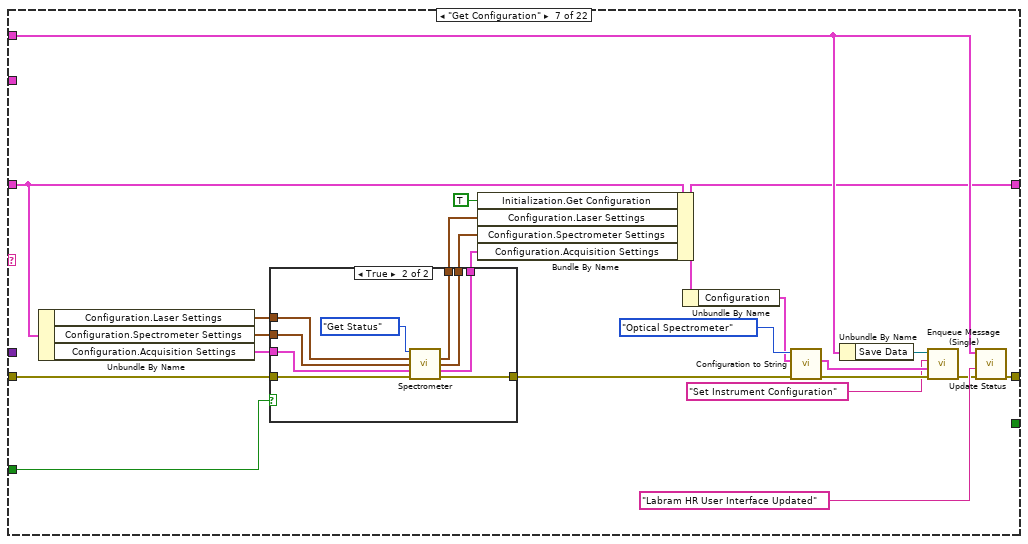
[diagram p11: hidden frame]
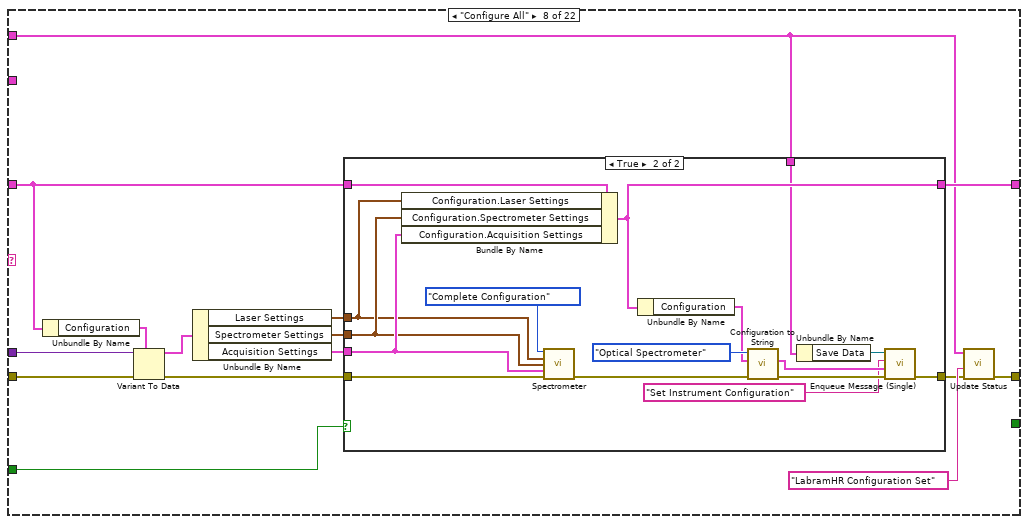
[diagram p13: hidden frame]
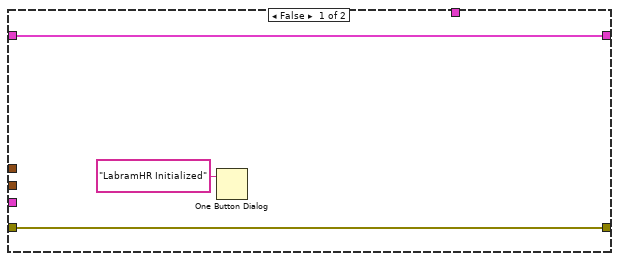
[diagram p14: hidden frame]
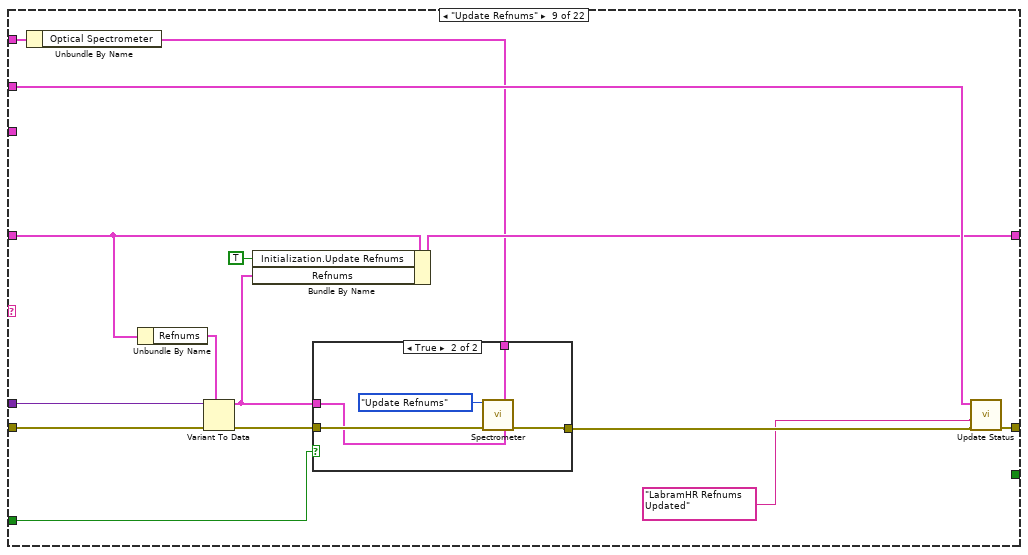
[diagram p15: hidden frame]
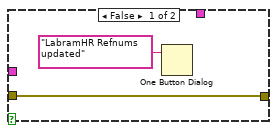
[diagram p16: hidden frame]
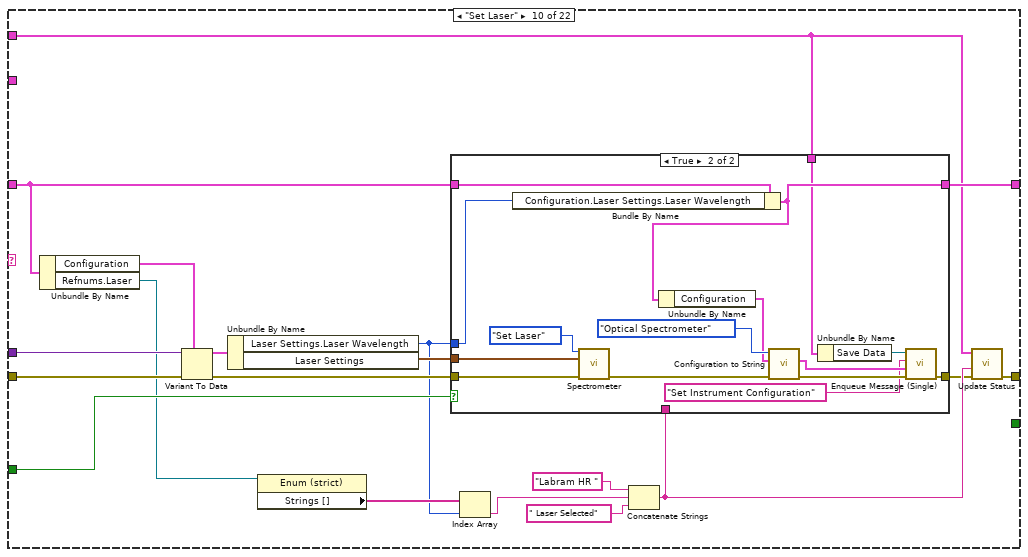
[diagram p17: hidden frame]
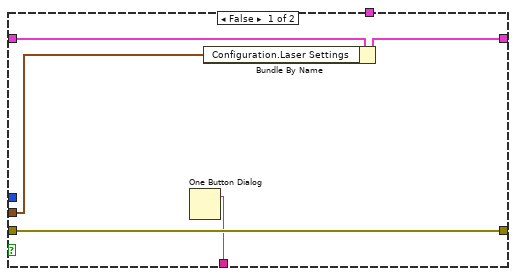
[diagram p18: hidden frame]
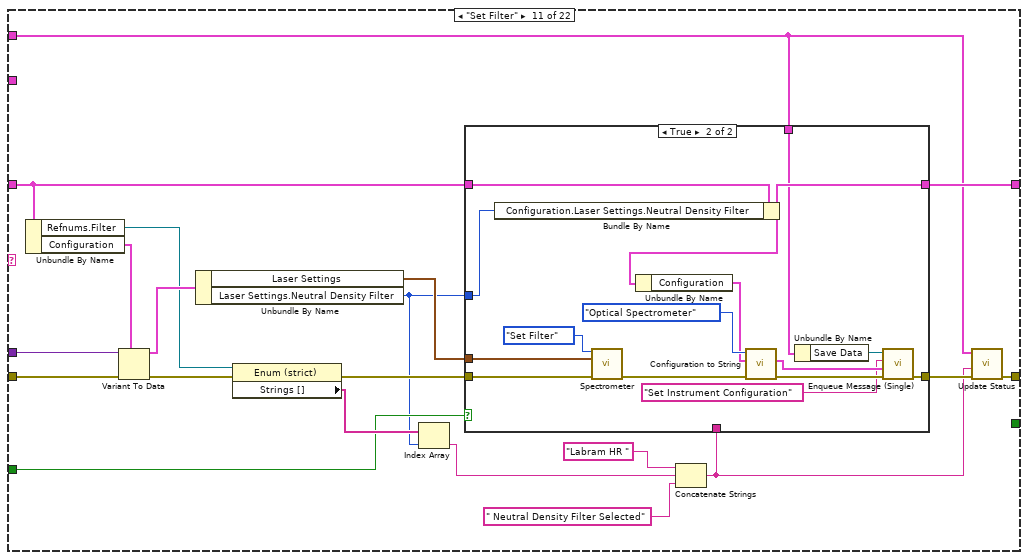
[diagram p19: hidden frame]
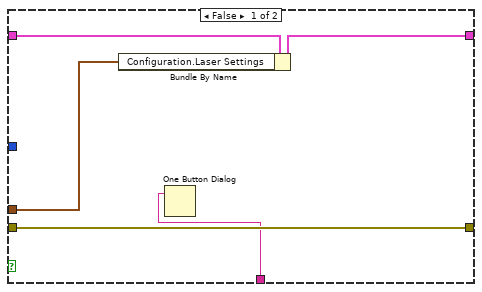
[diagram p20: hidden frame]
diagram:
  # "LICENSED MATERIALS – PROPERTY OF IBM\nCopyright IBM Corp. 2016,\nALL RIGHTS RESERVED"
  n1 = Unbundle By Name("Configuration") -> ("Optical Spectrometer"=w2:T12)
  n2 = call "Spectrometer Data.vi"() -> ("Spectrometer Data"=w1:T58)
  n3 = while "Queued Message Handler for Labram HR" {
    tunnel: "error in" -> [w21]
    tunnel: [w14] -> w4
    tunnel: "Message Queues out" -> [w17]
    tunnel: "Notifiers" -> [w8]
    tunnel: w2 -> [w11]
    shift-right: [w9] -> _
    shift-left: w1 -> [w10]
    stop <- w16 stop-if-true
    # "Configurations"
    # "Notifiers"
    # "Message Queues"
    n4 = Unbundle By Name(w17) -> ("Optical Spectrometer"=w13:refnum<queue>)
    n5 = call "Dequeue Message.vi"("error in (no error)"=w21, "Message Queue"=w13) -> ("error out"=w20:errorcluster, "Message Data"=w18:variant, "Message"=w19:string)  [unwired: 7 out]
    n6 = case shown="\"Error\"" w19 {
      selector: w19 -> [w24 _ _ _ _ _ _ _ _ _ _ _ _ _ _ _ _ _ _ _ _ _]
      tunnel: w20 -> [_ w35 w42 w63 w74 w93 w120 w147 w180 w208 w248 w285 w325 w364 w401 w433 w464 w496 w509 w528 w553 w570]
      tunnel: [w23 w34 w43 w54 w70 w85 w110 w137 w178 w204 w244 w278 w322 w362 w396 w430 w462 w491 w512 w536 w545 w569] -> w15
      tunnel: w18 -> [_ _ _ _ _ _ _ w145 w182 w206 w247 w283 w324 w363 w400 w434 w465 w489 _ _ _ _]
      tunnel: w17 -> [_ w33 w39 w62 w67 w88 w100 w134 w177 w191 w230 w270 w307 w347 w386 w422 w455 w497 w504 w527 w556 _]
      tunnel: w8 -> [_ _ _ w60 w66 _ _ _ w169 _ _ _ _ _ _ _ _ _ _ _ w549 w568]
      tunnel: [_ _ _ _ _ _ _ _ _ _ _ _ _ _ _ _ _ _ _ _ TRUE ("Priority Message? (F)") _] -> w16
      tunnel: w10 -> [w22 w32 w40 w55 w69 w91 w117 w136 w174 w192 w237 w272 w311 w353 w391 w427 w459 w488 w510 w534 w551 w566]
      tunnel: "Used functions" -> [_ _ _ _ _ w92 w119 w148 w179 w205 w233 w279 w308 w348 w387 w423 w456 _ w513 _ w554 _]
      tunnel: w11 -> [_ w29 _ _ _ _ _ _ _ _ _ _ _ _ _ _ _ _ _ _ _ _]
      tunnel: [w22 w30 w40 w55 w69 w90 w99 w135 w173 w193 w236 w271 w310 w352 w390 w426 w458 w488 w510 w534 w551 w566] -> w9
      frame Default {
        # "The Defualt Case run if there is a message that isn't defined in any of the other cases.\nOutput a program error"
        n7 = Format Into String(format string="The invalid message string \"%s\" was  received in the LabramHR Loop", w24) -> (resulting string=w26:string)  [unwired: 2 in, 1 out]
        n8 = call <vilib>:"Error Cluster From Error Code.vi"("error message (\"\")"=w26, "error code (0)"=5001) -> ("error out"=w23:errorcluster)  [unwired: 2 in, 5 out]
      }
      frame "Initialize" {
        # "No SetUI - Get Status from the Machine after Update Refnums"
        n9 = Unbundle By Name(w33) -> ("Optical Spectrometer"=w37:refnum<queue>, "Message Handler Loop"=w31:refnum<queue>)
        n10 = call "Enqueue Message (Single).vi"("error in (no error)"=w35, "Message"="LabramHR - Update Refnums", "Message Queue"=w31) -> ("error out"=w28:errorcluster)  [unwired: 1 in, 7 out]
        n11 = Bundle By Name(cluster=w32, "Configuration"=w29) -> (w30:T58)
        n12 = call "Enqueue Message (Single).vi"("error in (no error)"=w28, "Message"="Check if Refnums Updated", "Message Queue"=w37) -> ("error out"=w34:errorcluster)  [unwired: 1 in, 7 out]
      }
      frame "Check if Refnums Updated" {
        n13 = Unbundle By Name(w40) -> ("Initialization.Update Refnums"=w41:bool)
        n14 = case shown="True" w41 {
          tunnel: w39 -> [w48 w53]
          tunnel: w42 -> [w45 w50]
          tunnel: [w44 w49] -> w43
          frame False {
            n15 = Unbundle By Name(w48) -> ("Optical Spectrometer"=w47:refnum<queue>)
            n16 = call "Enqueue Message (Single).vi"("error in (no error)"=w45, "Message"="Check if Refnums Updated", "Message Queue"=w47) -> ("error out"=w44:errorcluster)  [unwired: 1 in, 7 out]
          }
          frame True {
            n17 = Unbundle By Name(w53) -> ("Optical Spectrometer"=w52:refnum<queue>)
            n18 = call "Enqueue Message (Single).vi"("error in (no error)"=w50, "Message"="Continue Initialize", "Message Queue"=w52) -> ("error out"=w49:errorcluster)  [unwired: 1 in, 7 out]
          }
        }
      }
      frame "Continue Initialize" {
        n19 = Unbundle By Name(w60) -> ("Save Data.Ready"=w59:refnum<notifier>)
        n20 = Wait on Notification(notifier=w59, error in (no error)=w63) -> (error out=w61:errorcluster)  [unwired: 2 in, 3 out]
        n21 = Unbundle By Name(w62) -> ("Optical Spectrometer"=w64:refnum<queue>)
        n22 = Build Array("Connect" ("Message"), "Get Configuration" ("Message"), "Ready" ("Message")) -> (w58:string[])
        n23 = call-poly "Enqueue Message.vi"("error in (no error)"=w61, "Message Array"=w58, "Message Queue"=w64) -> ("error out"=w54:errorcluster)  [unwired: 7 in, 1 out]
      }
      frame "Ready" {
        n24 = Unbundle By Name(w69) -> ("Initialization.Connect"=w72:bool, "Initialization.Update Refnums"=w71:bool, "Initialization.Get Configuration"=w68:bool)
        n25 = Compound Arithmetic op=AND(w72, w71, w68) -> (w73:bool)
        n26 = case shown="True" w73 {
          tunnel: [w78 w83] -> w70
          tunnel: w74 -> [w77 w82]
          tunnel: w67 -> [w76 _]
          tunnel: w66 -> [_ w80]
          frame False {
            n27 = Unbundle By Name(w76) -> ("Optical Spectrometer"=w75:refnum<queue>)
            n28 = call "Enqueue Message (Single).vi"("error in (no error)"=w77, "Message"="Ready", "Message Queue"=w75) -> ("error out"=w78:errorcluster)  [unwired: 1 in, 7 out]
          }
          frame True {
            n29 = Unbundle By Name(w80) -> ("Optical Spectrometer.Ready"=w81:refnum<notifier>)
            n30 = Send Notification(notification=TRUE, notifier=w81, error in (no error)=w82) -> (error out=w83:errorcluster)  [unwired: 1 out]
          }
        }
      }
      frame "Connect" {
        n31 = case shown="True" w92 {
          tunnel: w93 -> [w95 w98]
          tunnel: [w95 w97] -> w87
          frame False {
            n32 = One Button Dialog(message="LabramHR Connected" ("button name (\"OK\")")) -> ()  [unwired: 2 out]
          }
          frame True {
            n33 = call "Spectrometer.vi"("Function"=Spectrometer_Function."Connect", "error in"=w98) -> ("error out"=w97:errorcluster)  [unwired: 9 in, 4 out]
          }
        }
        n34 = Bundle By Name(cluster=w91, "Initialization.Connect"=TRUE) -> (w90:T58)
        n35 = call "Update Status.vi"("error in"=w87, "String"="Labram HR Connected", "Message Queues out"=w88) -> ("error out"=w85:errorcluster)  [unwired: 8 out]
      }
      frame "Get Configuration" {
        n36 = Unbundle By Name(w117) -> ("Configuration.Laser Settings"=w116:T13, "Configuration.Spectrometer Settings"=w114:T16, "Configuration.Acquisition Settings"=w115:T19)
        n37 = case shown="True" w119 {
          tunnel: w120 -> [w124 w133]
          tunnel: [w124 w125] -> w102
          tunnel: w116 -> [w123 w131]
          tunnel: w115 -> [w122 w130]
          tunnel: w114 -> [w121 w129]
          tunnel: [w123 w128] -> w113
          tunnel: [w122 w126] -> w112
          tunnel: [w121 w127] -> w111
          frame False {
          }
          frame True {
            n38 = call "Spectrometer.vi"("Function"=Spectrometer_Function."Get Status", "Laser Settings"=w131, "Spectrometer Settings"=w129, "Acquisition Settings"=w130, "error in"=w133) -> ("Laser Settings Out"=w128:T13, "Spectrometer Settings Out"=w127:T16, "Acquisition Settings Out"=w126:T19, "error out"=w125:errorcluster)  [unwired: 6 in, 1 out]
          }
        }
        n39 = Bundle By Name(cluster=w117, "Initialization.Get Configuration"=TRUE ("Initialization.Connect"), "Configuration.Laser Settings"=w113, "Configuration.Spectrometer Settings"=w111, "Configuration.Acquisition Settings"=w112) -> (w99:T58)
        n40 = Unbundle By Name(w99) -> ("Configuration"=w103:T12)
        n41 = call "Configuration to String.vi"("error in (no error)"=w102, "Configuration"=w103, "Instrument"=Instrument_List."Optical Spectrometer") -> ("error out"=w106:errorcluster, "Instrument Configuration"=w107:T33)  [unwired: 7 out]
        n42 = Unbundle By Name(w100) -> ("Save Data"=w105:refnum<queue>)
        n43 = call "Enqueue Message (Single).vi"("error in (no error)"=w106, "Message Data"=w107, "Message"="Set Instrument Configuration", "Message Queue"=w105) -> ("error out"=w101:errorcluster)  [unwired: 7 out]
        n44 = call "Update Status.vi"("error in"=w101, "String"="Labram HR User Interface Updated", "Message Queues out"=w100) -> ("error out"=w110:errorcluster)  [unwired: 8 out]
      }
      frame "Configure All" {
        n45 = Unbundle By Name(w136) -> ("Configuration"=w144:T12)
        n46 = Variant To Data(error in=w147, type=w144, Variant=w145) -> (data=w143:T12, error out=w146:errorcluster)
        n47 = Unbundle By Name(w143) -> ("Laser Settings"=w141:T13, "Spectrometer Settings"=w140:T16, "Acquisition Settings"=w142:T19)
        n48 = case shown="True" w148 {
          tunnel: [w151 w153] -> w138
          tunnel: w146 -> [w151 w167]
          tunnel: w142 -> [_ w164]
          tunnel: w141 -> [_ w162]
          tunnel: w140 -> [_ w163]
          tunnel: w136 -> [w149 w165]
          tunnel: [w149 w161] -> w135
          tunnel: w134 -> [_ w152]
          frame False {
            n49 = One Button Dialog(message="LabramHR Initialized" ("button name (\"OK\")")) -> ()  [unwired: 2 out]
          }
          frame True {
            n50 = Bundle By Name(cluster=w165, "Configuration.Laser Settings"=w162, "Configuration.Spectrometer Settings"=w163, "Configuration.Acquisition Settings"=w164) -> (w161:T58)
            n51 = call "Spectrometer.vi"("Function"=Spectrometer_Function."Complete Configuration", "Laser Settings"=w162, "Spectrometer Settings"=w163, "Acquisition Settings"=w164, "error in"=w167) -> ("error out"=w154:errorcluster)  [unwired: 6 in, 4 out]
            n52 = Unbundle By Name(w161) -> ("Configuration"=w155:T12)
            n53 = call "Configuration to String.vi"("error in (no error)"=w154, "Configuration"=w155, "Instrument"=Instrument_List."Optical Spectrometer") -> ("error out"=w158:errorcluster, "Instrument Configuration"=w159:T33)  [unwired: 7 out]
            n54 = Unbundle By Name(w152) -> ("Save Data"=w157:refnum<queue>)
            n55 = call "Enqueue Message (Single).vi"("error in (no error)"=w158, "Message Data"=w159, "Message"="Set Instrument Configuration", "Message Queue"=w157) -> ("error out"=w153:errorcluster)  [unwired: 7 out]
          }
        }
        n56 = call "Update Status.vi"("error in"=w138, "String"="LabramHR Configuration Set", "Message Queues out"=w134) -> ("error out"=w137:errorcluster)  [unwired: 8 out]
      }
      frame "Update Refnums" {
        n57 = Unbundle By Name(w169) -> ("Optical Spectrometer"=w168:T49)
        n58 = Unbundle By Name(w174) -> ("Refnums"=w172:T59)
        n59 = Variant To Data(error in=w180, type=w172, Variant=w182) -> (data=w171:T59, error out=w181:errorcluster)
        n60 = Bundle By Name(cluster=w174, "Initialization.Update Refnums"=TRUE, "Refnums"=w171) -> (w173:T58)
        n61 = case shown="True" w179 {
          tunnel: w171 -> [_ w186]
          tunnel: w181 -> [w184 w189]
          tunnel: [w184 w188] -> w176
          tunnel: w168 -> [_ w185]
          frame False {
            n62 = One Button Dialog(message="LabramHR Refnums updated" ("button name (\"OK\")")) -> ()  [unwired: 2 out]
          }
          frame True {
            n63 = call "Spectrometer.vi"("Function"=Spectrometer_Function."Update Refnums", "Labram HR Notifications"=w185, "error in"=w189, "LabramHR References"=w186) -> ("error out"=w188:errorcluster)  [unwired: 7 in, 4 out]
          }
        }
        n64 = call "Update Status.vi"("error in"=w176, "String"="LabramHR Refnums Updated" ("button name (\"OK\")"), "Message Queues out"=w177) -> ("error out"=w178:errorcluster)  [unwired: 8 out]
      }
      frame "Set Laser" {
        n65 = Unbundle By Name(w192) -> ("Configuration"=w200:T12, "Refnums.Laser"=w199:refnum<vi>)
        n66 = Variant To Data(error in=w208, type=w200, Variant=w206) -> (data=w201:T12, error out=w207:errorcluster)
        n67 = Unbundle By Name(w201) -> ("Laser Settings.Laser Wavelength"=w190:T14, "Laser Settings"=w195:T13)
        n68 = property class="Enum (strict)"(reference=w199) -> ("Strings []"=w197:string[])  [unwired: 1 in, 2 out]
        n69 = Index Array(array=w197, index=w190) -> (element=w196:string)
        n70 = Concatenate Strings("Labram HR " ("string"), w196, " Laser Selected" ("string")) -> (w203:string)
        n71 = case shown="True" w205 {
          tunnel: w207 -> [w213 w228]
          tunnel: [w213 w218] -> w202
          tunnel: w203 -> [w212 _]
          tunnel: w195 -> [w209 w225]
          tunnel: [w210 w216] -> w193
          tunnel: w192 -> [w211 w226]
          tunnel: w191 -> [_ w215]
          tunnel: w190 -> [_ w214]
          frame False {
            n72 = One Button Dialog(message=w212) -> ()  [unwired: 2 out]
            n73 = Bundle By Name(cluster=w211, "Configuration.Laser Settings"=w209) -> (w210:T58)
          }
          frame True {
            n74 = Bundle By Name(cluster=w226, "Configuration.Laser Settings.Laser Wavelength"=w214) -> (w216:T58)
            n75 = call "Spectrometer.vi"("Function"=Spectrometer_Function."Set Laser", "Laser Settings"=w225, "error in"=w228) -> ("error out"=w217:errorcluster)  [unwired: 8 in, 4 out]
            n76 = Unbundle By Name(w216) -> ("Configuration"=w219:T12)
            n77 = call "Configuration to String.vi"("error in (no error)"=w217, "Configuration"=w219, "Instrument"=Instrument_List."Optical Spectrometer") -> ("error out"=w222:errorcluster, "Instrument Configuration"=w223:T33)  [unwired: 7 out]
            n78 = Unbundle By Name(w215) -> ("Save Data"=w221:refnum<queue>)
            n79 = call "Enqueue Message (Single).vi"("error in (no error)"=w222, "Message Data"=w223, "Message"="Set Instrument Configuration", "Message Queue"=w221) -> ("error out"=w218:errorcluster)  [unwired: 7 out]
          }
        }
        n80 = call "Update Status.vi"("error in"=w202, "String"=w203, "Message Queues out"=w191) -> ("error out"=w204:errorcluster)  [unwired: 8 out]
      }
      frame "Set Filter" {
        n81 = Unbundle By Name(w237) -> ("Refnums.Filter"=w240:refnum<vi>, "Configuration"=w242:T12)
        n82 = Variant To Data(error in=w248, type=w242, Variant=w247) -> (data=w243:T12, error out=w239:errorcluster)
        n83 = Unbundle By Name(w243) -> ("Laser Settings"=w231:T13, "Laser Settings.Neutral Density Filter"=w229:T15)
        n84 = property class="Enum (strict)"(reference=w240, error in=w239) -> (error out=w234:errorcluster, "Strings []"=w241:string[])  [unwired: 1 out]
        n85 = Index Array(array=w241, index=w229) -> (element=w238:string)
        n86 = Concatenate Strings("Labram HR " ("string"), w238, " Neutral Density Filter Selected" ("string")) -> (w232:string)
        n87 = case shown="True" w233 {
          tunnel: w234 -> [w253 w268]
          tunnel: [w253 w258] -> w235
          tunnel: w232 -> [w252 _]
          tunnel: w231 -> [w250 w256]
          tunnel: w237 -> [w251 w266]
          tunnel: [w249 w257] -> w236
          tunnel: w230 -> [_ w255]
          tunnel: w229 -> [_ w254]
          frame False {
            n88 = Bundle By Name(cluster=w251, "Configuration.Laser Settings"=w250) -> (w249:T58)
            n89 = One Button Dialog(message=w252) -> ()  [unwired: 2 out]
          }
          frame True {
            n90 = Bundle By Name(cluster=w266, "Configuration.Laser Settings.Neutral Density Filter"=w254) -> (w257:T58)
            n91 = call "Spectrometer.vi"("Function"=Spectrometer_Function."Set Filter", "Laser Settings"=w256, "error in"=w268) -> ("error out"=w259:errorcluster)  [unwired: 8 in, 4 out]
            n92 = Unbundle By Name(w257) -> ("Configuration"=w260:T12)
            n93 = call "Configuration to String.vi"("error in (no error)"=w259, "Configuration"=w260, "Instrument"=Instrument_List."Optical Spectrometer") -> ("error out"=w263:errorcluster, "Instrument Configuration"=w264:T33)  [unwired: 7 out]
            n94 = Unbundle By Name(w255) -> ("Save Data"=w262:refnum<queue>)
            n95 = call "Enqueue Message (Single).vi"("error in (no error)"=w263, "Message Data"=w264, "Message"="Set Instrument Configuration", "Message Queue"=w262) -> ("error out"=w258:errorcluster)  [unwired: 7 out]
          }
        }
        n96 = call "Update Status.vi"("error in"=w235, "String"=w232, "Message Queues out"=w230) -> ("error out"=w244:errorcluster)  [unwired: 8 out]
      }
      frame "Set Hole" {
        n97 = Unbundle By Name(w272) -> ("Configuration"=w274:T12)
        n98 = Variant To Data(error in=w285, type=w274, Variant=w283) -> (data=w275:T12, error out=w284:errorcluster)
        n99 = Unbundle By Name(w275) -> ("Spectrometer Settings.Confocal Hole Size (µm)"=w269:dbl, "Spectrometer Settings"=w273:T16)
        n100 = Number To Decimal String(number=w269) -> (decimal integer string=w282:string)  [unwired: 1 out]
        n101 = Concatenate Strings("Labram HR  Confocal Hole Set To " ("string"), w282, " um" ("string")) -> (w276:string)
        n102 = case shown="True" w279 {
          tunnel: w284 -> [w290 w305]
          tunnel: [w290 w294] -> w277
          tunnel: w276 -> [w289 _]
          tunnel: w273 -> [w287 w302]
          tunnel: w272 -> [w288 w303]
          tunnel: [w286 w293] -> w271
          tunnel: w270 -> [_ w292]
          tunnel: w269 -> [_ w291]
          frame False {
            n103 = Bundle By Name(cluster=w288, "Configuration.Spectrometer Settings"=w287) -> (w286:T58)
            n104 = One Button Dialog(message=w289) -> ()  [unwired: 2 out]
          }
          frame True {
            n105 = Bundle By Name(cluster=w303, "Configuration.Spectrometer Settings.Confocal Hole Size (µm)"=w291) -> (w293:T58)
            n106 = call "Spectrometer.vi"("Function"=Spectrometer_Function."Set Hole", "Spectrometer Settings"=w302, "error in"=w305) -> ("error out"=w295:errorcluster)  [unwired: 8 in, 4 out]
            n107 = Unbundle By Name(w293) -> ("Configuration"=w296:T12)
            n108 = call "Configuration to String.vi"("error in (no error)"=w295, "Configuration"=w296, "Instrument"=Instrument_List."Optical Spectrometer") -> ("error out"=w299:errorcluster, "Instrument Configuration"=w300:T33)  [unwired: 7 out]
            n109 = Unbundle By Name(w292) -> ("Save Data"=w298:refnum<queue>)
            n110 = call "Enqueue Message (Single).vi"("error in (no error)"=w299, "Message Data"=w300, "Message"="Set Instrument Configuration", "Message Queue"=w298) -> ("error out"=w294:errorcluster)  [unwired: 7 out]
          }
        }
        n111 = call "Update Status.vi"("error in"=w277, "String"=w276, "Message Queues out"=w270) -> ("error out"=w278:errorcluster)  [unwired: 8 out]
      }
      frame "Set Grating" {
        n112 = Unbundle By Name(w311) -> ("Configuration"=w321:T12, "Refnums.Grating"=w318:refnum<vi>)
        n113 = Variant To Data(error in=w325, type=w321, Variant=w324) -> (data=w320:T12, error out=w315:errorcluster)
        n114 = Unbundle By Name(w320) -> ("Spectrometer Settings"=w312:T16, "Spectrometer Settings.Grating"=w306:T17)
        n115 = property class="Ring (strict)"(reference=w318, error in=w315) -> (error out=w313:errorcluster, "Strings []"=w317:string[])  [unwired: 1 out]
        n116 = Index Array(array=w317, index=w306) -> (element=w316:string)
        n117 = Concatenate Strings("Labram HR " ("string"), w316, " Grating Selected" ("string")) -> (w314:string)
        n118 = case shown="True" w308 {
          tunnel: w313 -> [w330 w345]
          tunnel: [w330 w334] -> w309
          tunnel: w314 -> [w329 _]
          tunnel: w312 -> [w327 w342]
          tunnel: w311 -> [w328 w343]
          tunnel: [w326 w333] -> w310
          tunnel: w307 -> [_ w332]
          tunnel: w306 -> [_ w331]
          frame False {
            n119 = Bundle By Name(cluster=w328, "Configuration.Spectrometer Settings"=w327) -> (w326:T58)
            n120 = One Button Dialog(message=w329) -> ()  [unwired: 2 out]
          }
          frame True {
            n121 = Bundle By Name(cluster=w343, "Configuration.Spectrometer Settings.Grating"=w331) -> (w333:T58)
            n122 = call "Spectrometer.vi"("Function"=Spectrometer_Function."Set Grating", "Spectrometer Settings"=w342, "error in"=w345) -> ("error out"=w335:errorcluster)  [unwired: 8 in, 4 out]
            n123 = Unbundle By Name(w333) -> ("Configuration"=w336:T12)
            n124 = call "Configuration to String.vi"("error in (no error)"=w335, "Configuration"=w336, "Instrument"=Instrument_List."Optical Spectrometer") -> ("error out"=w339:errorcluster, "Instrument Configuration"=w340:T33)  [unwired: 7 out]
            n125 = Unbundle By Name(w332) -> ("Save Data"=w338:refnum<queue>)
            n126 = call "Enqueue Message (Single).vi"("error in (no error)"=w339, "Message Data"=w340, "Message"="Set Instrument Configuration", "Message Queue"=w338) -> ("error out"=w334:errorcluster)  [unwired: 7 out]
          }
        }
        n127 = call "Update Status.vi"("error in"=w309, "String"=w314, "Message Queues out"=w307) -> ("error out"=w322:errorcluster)  [unwired: 8 out]
      }
      frame "Set Detector" {
        n128 = Unbundle By Name(w353) -> ("Configuration"=w361:T12, "Refnums.Detector"=w358:refnum<vi>)
        n129 = Variant To Data(error in=w364, type=w361, Variant=w363) -> (data=w360:T12, error out=w355:errorcluster)
        n130 = Unbundle By Name(w360) -> ("Spectrometer Settings"=w351:T16, "Spectrometer Settings.Detector"=w346:T18)
        n131 = property class="Enum (strict)"(reference=w358, error in=w355) -> (error out=w350:errorcluster, "Strings []"=w357:string[])  [unwired: 1 out]
        n132 = Index Array(array=w357, index=w346) -> (element=w356:string)
        n133 = Concatenate Strings("Labram HR Acquisition with " ("string"), w356) -> (w349:string)
        n134 = case shown="True" w348 {
          tunnel: [w365 w376] -> w354
          tunnel: [w369 w375] -> w352
          tunnel: w353 -> [w368 w374]
          tunnel: w351 -> [w367 w373]
          tunnel: w350 -> [w365 w372]
          tunnel: w349 -> [w366 _]
          tunnel: w347 -> [_ w371]
          tunnel: w346 -> [_ w370]
          frame False {
            n135 = Bundle By Name(cluster=w368, "Configuration.Spectrometer Settings"=w367) -> (w369:T58)
            n136 = One Button Dialog(message=w366) -> ()  [unwired: 2 out]
          }
          frame True {
            n137 = Bundle By Name(cluster=w374, "Configuration.Spectrometer Settings.Detector"=w370) -> (w375:T58)
            n138 = Unbundle By Name(w375) -> ("Configuration"=w378:T12)
            n139 = call "Spectrometer.vi"("Function"=Spectrometer_Function."Set Detector", "Spectrometer Settings"=w373, "error in"=w372) -> ("error out"=w377:errorcluster)  [unwired: 8 in, 4 out]
            n140 = call "Configuration to String.vi"("error in (no error)"=w377, "Configuration"=w378, "Instrument"=Instrument_List."Optical Spectrometer") -> ("error out"=w381:errorcluster, "Instrument Configuration"=w382:T33)  [unwired: 7 out]
            n141 = Unbundle By Name(w371) -> ("Save Data"=w380:refnum<queue>)
            n142 = call "Enqueue Message (Single).vi"("error in (no error)"=w381, "Message Data"=w382, "Message"="Set Instrument Configuration", "Message Queue"=w380) -> ("error out"=w376:errorcluster)  [unwired: 7 out]
          }
        }
        n143 = call "Update Status.vi"("error in"=w354, "String"=w349, "Message Queues out"=w347) -> ("error out"=w362:errorcluster)  [unwired: 8 out]
      }
      frame "Set Spectal Position" {
        n144 = Unbundle By Name(w391) -> ("Configuration"=w394:T12)
        n145 = Variant To Data(error in=w401, type=w394, Variant=w400) -> (data=w395:T12, error out=w388:errorcluster)
        n146 = Unbundle By Name(w395) -> ("Acquisition Settings"=w389:T19, "Acquisition Settings.Spectal Position (nm)"=w385:dbl)
        n147 = Number To Decimal String(number=w385) -> (decimal integer string=w399:string)  [unwired: 1 out]
        n148 = Concatenate Strings("Labram HR Grating Position Set To " ("string"), w399, " nm" ("string")) -> (w392:string)
        n149 = case shown="True" w387 {
          tunnel: [w402 w414] -> w393
          tunnel: [w406 w411] -> w390
          tunnel: w392 -> [w405 _]
          tunnel: w391 -> [w404 w412]
          tunnel: w389 -> [w403 w408]
          tunnel: w388 -> [w402 w413]
          tunnel: w386 -> [_ w410]
          tunnel: w385 -> [_ w407]
          frame False {
            n150 = Bundle By Name(cluster=w404, "Configuration.Acquisition Settings"=w403) -> (w406:T58)
            n151 = One Button Dialog(message=w405) -> ()  [unwired: 2 out]
          }
          frame True {
            n152 = Bundle By Name(cluster=w412, "Configuration.Acquisition Settings.Spectal Position (nm)"=w407) -> (w411:T58)
            n153 = call "Spectrometer.vi"("Function"=Spectrometer_Function."Set Grating Position", "Acquisition Settings"=w408, "error in"=w413) -> ("error out"=w409:errorcluster)  [unwired: 8 in, 4 out]
            n154 = Unbundle By Name(w411) -> ("Configuration"=w415:T12)
            n155 = call "Configuration to String.vi"("error in (no error)"=w409, "Configuration"=w415, "Instrument"=Instrument_List."Optical Spectrometer") -> ("error out"=w418:errorcluster, "Instrument Configuration"=w419:T33)  [unwired: 7 out]
            n156 = Unbundle By Name(w410) -> ("Save Data"=w417:refnum<queue>)
            n157 = call "Enqueue Message (Single).vi"("error in (no error)"=w418, "Message Data"=w419, "Message"="Set Instrument Configuration", "Message Queue"=w417) -> ("error out"=w414:errorcluster)  [unwired: 7 out]
          }
        }
        n158 = call "Update Status.vi"("error in"=w393, "String"=w392, "Message Queues out"=w386) -> ("error out"=w396:errorcluster)  [unwired: 8 out]
      }
      frame "Set Acquisition Settings" {
        w428 = "Labram HR Acquisition Settings Updated" ("String")
        n159 = Unbundle By Name(w427) -> ("Configuration"=w431:T12)
        n160 = Variant To Data(error in=w433, type=w431, Variant=w434) -> (data=w432:T12, error out=w429:errorcluster)
        n161 = Unbundle By Name(w432) -> ("Acquisition Settings"=w425:T19)
        n162 = case shown="True" w423 {
          tunnel: [w435 w445] -> w424
          tunnel: [w439 w441] -> w426
          tunnel: w428 -> [w438 _]
          tunnel: w427 -> [w437 w443]
          tunnel: w425 -> [w436 w442]
          tunnel: w429 -> [w435 w444]
          tunnel: w422 -> [_ w440]
          frame False {
            n163 = Bundle By Name(cluster=w437, "Configuration.Acquisition Settings"=w436) -> (w439:T58)
            n164 = One Button Dialog(message=w438) -> ()  [unwired: 2 out]
          }
          frame True {
            n165 = Bundle By Name(cluster=w443, "Configuration.Acquisition Settings"=w442) -> (w441:T58)
            n166 = call "Spectrometer.vi"("Function"=Spectrometer_Function."Set Acquisition Mode", "Acquisition Settings"=w442, "error in"=w444) -> ("error out"=w446:errorcluster)  [unwired: 8 in, 4 out]
            n167 = Unbundle By Name(w441) -> ("Configuration"=w447:T12)
            n168 = call "Configuration to String.vi"("error in (no error)"=w446, "Configuration"=w447, "Instrument"=Instrument_List."Optical Spectrometer") -> ("error out"=w450:errorcluster, "Instrument Configuration"=w451:T33)  [unwired: 7 out]
            n169 = Unbundle By Name(w440) -> ("Save Data"=w449:refnum<queue>)
            n170 = call "Enqueue Message (Single).vi"("error in (no error)"=w450, "Message Data"=w451, "Message"="Set Instrument Configuration", "Message Queue"=w449) -> ("error out"=w445:errorcluster)  [unwired: 7 out]
          }
        }
        n171 = call "Update Status.vi"("error in"=w424, "String"=w428, "Message Queues out"=w422) -> ("error out"=w430:errorcluster)  [unwired: 8 out]
      }
      frame "Complete Configuration" {
        w460 = "Labram HR Configured" ("String")
        n172 = Unbundle By Name(w459) -> ("Configuration"=w463:T12)
        n173 = Variant To Data(error in=w464, type=w463, Variant=w465) -> (data=w454:T12, error out=w461:errorcluster)
        n174 = case shown="True" w456 {
          tunnel: [w466 w479] -> w457
          tunnel: [w470 w476] -> w458
          tunnel: w460 -> [w469 _]
          tunnel: w459 -> [w468 w477]
          tunnel: w454 -> [w467 w474]
          tunnel: w461 -> [w466 w478]
          tunnel: w455 -> [_ w475]
          frame False {
            n175 = Bundle By Name(cluster=w468, "Configuration"=w467) -> (w470:T58)
            n176 = One Button Dialog(message=w469) -> ()  [unwired: 2 out]
          }
          frame True {
            n177 = Unbundle By Name(w474) -> ("Laser Settings"=w471:T13, "Spectrometer Settings"=w472:T16, "Acquisition Settings"=w473:T19)
            n178 = Bundle By Name(cluster=w477, "Configuration"=w474) -> (w476:T58)
            n179 = call "Spectrometer.vi"("Function"=Spectrometer_Function."Complete Configuration", "Laser Settings"=w471, "Spectrometer Settings"=w472, "Acquisition Settings"=w473, "error in"=w478) -> ("error out"=w480:errorcluster)  [unwired: 6 in, 4 out]
            n180 = Unbundle By Name(w476) -> ("Configuration"=w481:T12)
            n181 = call "Configuration to String.vi"("error in (no error)"=w480, "Configuration"=w481, "Instrument"=Instrument_List."Optical Spectrometer") -> ("error out"=w484:errorcluster, "Instrument Configuration"=w485:T33)  [unwired: 7 out]
            n182 = Unbundle By Name(w475) -> ("Save Data"=w483:refnum<queue>)
            n183 = call "Enqueue Message (Single).vi"("error in (no error)"=w484, "Message Data"=w485, "Message"="Set Instrument Configuration", "Message Queue"=w483) -> ("error out"=w479:errorcluster)  [unwired: 7 out]
          }
        }
        n184 = call "Update Status.vi"("error in"=w457, "String"=w460, "Message Queues out"=w455) -> ("error out"=w462:errorcluster)  [unwired: 8 out]
      }
      frame "Error" {
        # "Clear Errors to avoid getting stuck \nin repeating this case"
        # "Add here Cases that are handled \nalready by the Message Handler Loop"
        n185 = Variant To Data(error in=w496, type=errorcluster {"status"=FALSE, "code"=0, "source"=""} ("error out"), Variant=w489) -> (data=w495:errorcluster, error out=w494:errorcluster)
        n186 = Merge Errors(w495, w494) -> (w493:errorcluster)
        n187 = Unbundle By Name(w497) -> ("Message Handler Loop"=w499:refnum<queue>)
        n188 = Unbundle By Name(w493) -> ("code"=w490:i32)
        n189 = case shown="Default" w490 {
          tunnel: w499 -> [w503]
          tunnel: w493 -> [w501]
          tunnel: [w500] -> w492
          frame Default {
            n190 = call "Enqueue Message (Single).vi"("Message Data"=w501, "Message"="Error", "Message Queue"=w503) -> ("error out"=w500:errorcluster)  [unwired: 1 in, 7 out]
          }
        }
        n191 = call <vilib>:"Clear Errors.vi"("error in (no error)"=w492) -> ("error out"=w491:errorcluster)  [unwired: 1 in, 5 out]
      }
      frame "Acquire Spectrum" {
        n192 = Unbundle By Name(w510) -> ("Configuration.Laser Settings"=w505:T13, "Configuration.Spectrometer Settings"=w506:T16, "Configuration.Acquisition Settings"=w507:T19)
        n193 = case shown="True" w513 {
          tunnel: [w514 w519] -> w508
          tunnel: w509 -> [w514 w526]
          tunnel: w507 -> [_ w524]
          tunnel: w506 -> [_ w523]
          tunnel: w505 -> [_ w522]
          tunnel: w504 -> [_ w518]
          frame False {
            n194 = One Button Dialog(message="Acquisition" ("button name (\"OK\")")) -> ()  [unwired: 2 out]
          }
          frame True {
            n195 = call "Spectrometer.vi"("Function"=Spectrometer_Function."Acquire Spectrum", "Laser Settings"=w522, "Spectrometer Settings"=w523, "Acquisition Settings"=w524, "error in"=w526) -> ("Spectrum"=w516:T35, "error out"=w517:errorcluster)  [unwired: 6 in, 3 out]
            n196 = Unbundle By Name(w518) -> ("Save Data"=w521:refnum<queue>)
            n197 = call "Enqueue Message (Single).vi"("error in (no error)"=w517, "Message Data"=w516, "Message"="Set Optical Spectrum", "Message Queue"=w521) -> ("error out"=w519:errorcluster)  [unwired: 7 out]
          }
        }
        n198 = call "Update Status.vi"("error in"=w508, "String"="Labram HR Spectrum acquired" ("Message"), "Message Queues out"=w504) -> ("error out"=w512:errorcluster)  [unwired: 8 out]
      }
      frame "Save Optical Spectrum" {
        n199 = call "Set Device Information.vi"() -> ("error out"=w531:errorcluster, "Workspace Info"=w530:T32, "OK?"=w533:bool)  [unwired: 1 in, 8 out]
        n200 = Merge Errors(w531, w528) -> (w532:errorcluster)
        n201 = case shown="True" w533 {
          tunnel: w532 -> [w537 w542]
          tunnel: [w537 w541] -> w529
          tunnel: w530 -> [_ w540]
          tunnel: w527 -> [_ w539]
          frame False {
          }
          frame True {
            n202 = Unbundle By Name(w539) -> ("Save Data"=w538:refnum<queue>)
            n203 = call "Enqueue Message (Single).vi"("error in (no error)"=w542, "Message Data"=w540, "Message"="Save Optical Spectrum", "Message Queue"=w538) -> ("error out"=w541:errorcluster)  [unwired: 7 out]
          }
        }
        n204 = call "Update Status.vi"("error in"=w529, "String"="Labram HR Spectrum Saved" ("Message"), "Message Queues out"=w527) -> ("error out"=w536:errorcluster)  [unwired: 8 out]
      }
      frame "Exit" {
        w546 = TRUE ("Priority Message? (F)")
        # "Stop the VI"
        n205 = case shown="True" w554 {
          tunnel: w553 -> [w561 w565]
          tunnel: [w560 w564] -> w552
          tunnel: w549 -> [w559 _]
          frame False {
            n206 = Unbundle By Name(w559) -> ("Optical Spectrometer.Status"=w558:refnum<notifier>)
            n207 = Send Notification(notification="Disconnected", notifier=w558, error in (no error)=w561) -> (error out=w560:errorcluster)  [unwired: 1 out]
          }
          frame True {
            n208 = call "Spectrometer.vi"("Function"=Spectrometer_Function."Disconnect", "error in"=w565) -> ("error out"=w564:errorcluster)  [unwired: 9 in, 4 out]
          }
        }
        n209 = Unbundle By Name(w556) -> ("Optical Spectrometer"=w557:refnum<queue>)
        n210 = Unbundle By Name(w549) -> ("Optical Spectrometer.Ready"=w544:refnum<notifier>, "Optical Spectrometer.Exit"=w550:refnum<notifier>)
        n211 = Release Queue(queue=w557, error in (no error)=w552) -> (error out=w555:errorcluster)  [unwired: 3 out]
        n212 = Send Notification(notification=w546, notifier=w550, error in (no error)=w555) -> (error out=w547:errorcluster)  [unwired: 1 out]
        n213 = Send Notification(notification=w546, notifier=w544, error in (no error)=w547) -> (error out=w545:errorcluster)  [unwired: 1 out]
      }
      frame "Notify Status" {
        n214 = Unbundle By Name(w568) -> ("Optical Spectrometer.Instrument Data"=w567:refnum<notifier>)
        n215 = Send Notification(notification=w566, notifier=w567, error in (no error)=w570) -> (error out=w569:errorcluster)  [unwired: 1 out]
      }
    }
    n216 = call "Message Handling Loop.vi"("error in (no error)"=w15, "Message Queue"=w13) -> ("dup error in"=w14:errorcluster)  [unwired: 9 out]
  }
  "error out" <- w4
